vi "BStAT_(Singles).vi"() -> ()   [LabVIEW 2013]
uses:
  <vilib>/Utility/miscctls.llb/LVPositionTypeDef.ctl
  <vilib>/Utility/file.llb/Read From Spreadsheet File (DBL).vi
  <vilib>/Utility/file.llb/Write To Spreadsheet File (I64).vi
panel:
  out "framesPerSecond":u32
  out "serve to point":dbl[](array[numeric])
  in  "Word._Application":refnum<k7>
  out "p2y":dbl[](array[numeric])
  out "p1y":dbl[](array[numeric])
  out "point frames":dbl[](array[numeric])
  out "service frames":dbl[](array[numeric])
  out "comp_p1 2":dbl[](array[numeric])
  out "comp_p2 2":dbl[](array[numeric])
  out "comp_p2":dbl[](array[numeric])
  out "comp_p1":dbl[](array[numeric])
  out "game":i32[][](array[numeric])
  out "save2_data":dbl[][](array[numeric])
  out "save1_data":dbl[][](array[numeric])
  out "save2":i32[][](array[numeric])
  out "save1":i32[][](array[numeric])
  out "filedata in":dbl[][](array[numeric]) format="%0.3f"
  out "edited\nevents":dbl[][](array[numeric])
  out "edited to play":dbl[](array[numeric])
  out "P2 position":bool
  out "P1 position":bool
  out "p2code":i32
  out "p1code":i32
  out "frames":dbl[](array[numeric])
  out "Events":bool[](array[boolean])
  out "coded data":dbl[][](array[numeric])
  out "frame data":dbl[][](array[numeric])
  out "Score":dbl[][](array[numeric])
  out "OH":bool[](array[boolean])
  out "BH":bool[](array[boolean])
  out "FH":bool[](array[boolean])
  in  "stop":bool
  in  "Tab Control":enum32{"Coding", "Display"}(tab)
  in  "Drag control":u32(slide) min=400 max=3000 scale=0.0..37378.0
  in  "UNDO":bool
  out "Last coded":i32
  in  "Progress...":i32(slide) min=400 max=3000 scale=0.0..36584.0
  in  "1":bool
  in  "E2":bool
  in  "E1":bool
  in  "P2":i32
  in  "W2":bool
  in  "W1":bool
  in  "P1":i32
  in  "Pause 2":bool
  in  "F_Fr":bool
  in  "S_Fr":bool
  out "Video":T1(plugin-control)
  in  "START":bool
  in  "Video file":path caption="Open AVI file"
  in  "Save data":path caption="Save data to file"
  in  "Start Coding":bool
  out "F_frame":u32
  out "S_frame":u32
  in  "playback speed":dbl(slide) step=0.25 scale=0.25..2.0
  in  "fast forward":bool
  in  "TL 2":bool
  in  "BR 2":bool
  in  "BL 2":bool
  in  "BM 2":bool
  in  "CR  2":bool
  in  "CM 2":bool
  in  "CL 2":bool
  in  "TR 2":bool
  in  "TM 2":bool
  in  "TL 3":bool
  in  "BR 3":bool
  in  "BL 3":bool
  in  "BM 3":bool
  in  "CR  3":bool
  in  "CM 3":bool
  in  "CL 3":bool
  in  "TR 3":bool
  in  "TM 3":bool
  in  "Pause 1":bool
  out "coding":i32[][](array[numeric])
  in  "1 6":bool
  in  "2 6":bool
  in  "3 6":bool
  in  "4 6":bool
  in  "5 6":bool
  in  "6 6":bool
  in  "7 6":bool
  in  "8 6":bool
  in  "1 5":bool
  in  "2 5":bool
  in  "3 5":bool
  in  "4 5":bool
  in  "5 5":bool
  in  "6 5":bool
  in  "7 5":bool
  in  "8 5":bool
  in  "8 3":bool
  in  "7 3":bool
  in  "6 3":bool
  in  "5 3":bool
  in  "4 3":bool
  in  "3 3":bool
  in  "2 3":bool
  in  "1 3":bool
  in  "8 4":bool
  in  "7 4":bool
  in  "6 4":bool
  in  "5 4":bool
  in  "4 4":bool
  in  "3 4":bool
  in  "2 4":bool
  in  "1 4":bool
  in  "1 2":bool
  in  "2 2":bool
  in  "3 2":bool
  in  "4 2":bool
  in  "5 2":bool
  in  "6 2":bool
  in  "7 2":bool
  in  "8 2":bool
  in  "5":bool
  in  "6":bool
  in  "7":bool
  in  "8":bool
  in  "1":bool
  in  "2":bool
  in  "3":bool
  in  "4":bool
  in  "S2":bool
  in  "S1":bool
  in  "2":bool
  in  "3":bool
  in  "4":bool
  in  "Pause 3":bool
  in  "court":bool
  in  "Stop and save":bool
  out "Numeric":dbl format="%<%H:%M:%S>t"
  in  "play back":i32(slide)=1 min=0 max=7 scale=0.0..7.0
  out "DISP":T1(plugin-control)
  in  "Vid file":path caption="Open AVI file"
  in  "Data file":path caption="Read data from"
  in  "Tab Control 2":enum32{"Edit ", "Data Display", "Momentum"}(tab)
  in  "shots":u8(slide)=2 scale=0.0..5.0
  in  "point 2":bool
  in  "Rally":bool
  in  "Write VI":path caption="Write to AVI file"
  in  "before":u8(slide)=2
  in  "Playback Speed":dbl(slide)=1.0 min=0.25 max=30.0 step=0.25 scale=0.25..2.0
  in  "pause":bool
  in  "stop 2":bool
  in  "Playback\nscore":bool
  in  "P2 score":dbl
  in  "P1 score":dbl
  in  "error":bool
  in  "winner":bool
  in  "point 1":bool
  in  "player1":bool
  in  "player2":bool
  in  "1 7":bool
  in  "service2":bool
  in  "service1":bool
  in  "2 7":bool
  in  "3 7":bool
  in  "4 7":bool
  in  "TL":bool
  in  "BR":bool
  in  "BL":bool
  in  "BM":bool
  in  "CR":bool
  in  "CM":bool
  in  "CL":bool
  in  "TR":bool
  in  "TM":bool
  in  "FH 2":bool
  in  "BH 2":bool
  in  "ST":bool
  in  "CR 2":bool
  in  "lob":bool
  in  "clear":bool
  in  "drive":bool
  in  "smash":bool
  in  "defense":bool
  in  "chop":bool
  in  "drop":bool
  in  "net":bool
  in  "OH 2":bool
  in  "Play":bool
  in  "after":u8(slide)=2 scale=0.0..5.0
  in  "write file":bool
  out "Search events":i32(slide) caption="Scaning(events)..." min=400 max=3000 scale=0.0..903.0
  out "Search score":i32(slide) caption="Searching(score)..." min=400 max=3000 scale=0.0..1.0
  out "writing":i32(slide) caption="Writing..." min=400 max=3000 scale=0.0..7.0
  in  "3 shots":bool
  in  "Compare":bool
  in  "2":string(combo)="1"
  in  "1":string(combo)="1"
  in  "save2":string
  in  "save1":string
  in  "save2":bool
  in  "save1":bool
  in  "Percentage":bool
  in  "display\nselection":string(combo)="1"
  in  "To make white":enum32{""}(tab)
  out "player1 2":string[](array[string])
  out "player2 2":string[](array[string])
  out "P1graph":cluster{dbl[], "array":dbl[]}(graph)={[0.0, nan, 0.0, nan, 0.0, nan, 0.0, nan, 0.0, nan, 0.0, nan, 0.0, nan, 0.0, nan, 0.0], "array"=[1.0, 2.0, 3.0, 4.0, 5.0, 6.0, 7.0, 8.0, 9.0, 10.0, 11.0, 12.0, 13.0, 14.0, 15.0, 16.0, 17.0]}
  out "P2graph":cluster{dbl[], "array":dbl[]}(graph)={[0.0, nan, 0.0, nan, 0.0, nan, 0.0, nan, 0.0, nan, 0.0, nan, 0.0, nan, 0.0, nan, 0.0], "array"=[1.0, 2.0, 3.0, 4.0, 5.0, 6.0, 7.0, 8.0, 9.0, 10.0, 11.0, 12.0, 13.0, 14.0, 15.0, 16.0, 17.0]}
  out "W1/E1":string[](array[string])
  out "W2/E2":string[](array[string])
  out "W/E2":string[](array[string])=["Fore hand", "Back hand", "Over head", "", "Strainght", "Cross", "", "Lob", "Clear", "Drive", "Smash", "Defence", "Chop", "Drop", "Net"]
  out "W/E1":string[](array[string])=["Fore hand", "Back hand", "Over head", "", "Strainght", "Cross", "", "Lob", "Clear", "Drive", "Smash", "Defence", "Chop", "Drop", "Net"]
  out "player2_2":string[](array[string])
  out "player1_2":string[](array[string])
  out "Player 2":string[](array[string])=["Fore hand", "Back hand", "Over head", "", "Straight", "Cross", "", "Smash", "Defense", "Drive/Tap", "Lob", "Drop", "Chop", "Clear", "Net"]
  out "Player 2_2":string[](array[string])=["Fore hand", "Back hand", "Over head", "", "Strainght", "Cross", "", "Lob", "Clear", "Drive", "Smash", "Defence", "Chop", "Drop", "Net"]
  out "Player 1_2":string[](array[string])=["Fore hand", "Back hand", "Over head", "", "Strainght", "Cross", "", "Lob", "Clear", "Drive", "Smash", "Defence", "Chop", "Drop", "Net"]
  out "Player 1":string[](array[string])=["Fore hand", "Back hand", "Over head", "", "Straight", "Cross", "", "Smash", "Defense", "Drive/Tap", "Lob", "Drop", "Chop", "Clear", "Net"]
  out "p2 17":string
  out "p2 16":string
  out "p2 11":string
  out "p2 10":string
  out "p2 9":string
  out "p2 14":string
  out "p2 13":string
  out "p2 12":string
  out "p2 15":string
  out "p1 5":string
  out "p1 7":string
  out "p1 6":string
  out "p1 4":string
  out "p1 1":string
  out "p1 3":string
  out "p1 2":string
  out "p1 8":string
  out "p1 9":string
  in  "to make white 2":enum32{""}(tab)
  out "Shortest rally length(sec)":dbl format="%#_3g"
  out "Longest rally length(sec)":dbl format="%#_3g"
  out "momentum graph":cluster{dbl[], dbl[]}[](graph)
  out "Score":dbl[](array[numeric])
  out "Average rally length(sec)":dbl format="%#_3g"
  out "Rally length(sec)":dbl format="%#_3g"
  in  "edit video":bool
  in  "REPORT":bool
  # "Strategic Analysis Tool for Badminton"
  # "Forehand"
  # "Backhand"
  # "Overhead"
  # "Position"
  # "Straight"
  # "Cross"
  # "Straight"
  # "Cross"
  # "Straight"
  # "Cross"
  # "Smash"
  # "Defence"
  # "Drive/Tap"
  # "Lob"
  # "Drop"
  # "Chop"
  # "Player 2\n\nPlayer 1"
  # "Player 1\n\nPlayer 2"
  # "Clear"
  # "Net"
  # "Score"
  # "© 2012 National Sports Institute of Malaysia All Rights Reserved"
  # "© 2012 National Sports Institute of Malaysia All Rights Reserved"
  # "Shots to Playback"
  # "Score"
  # "Player"
  # "Position"
  # "Special Events"
  # "Playback interval (s)"
  # "to"
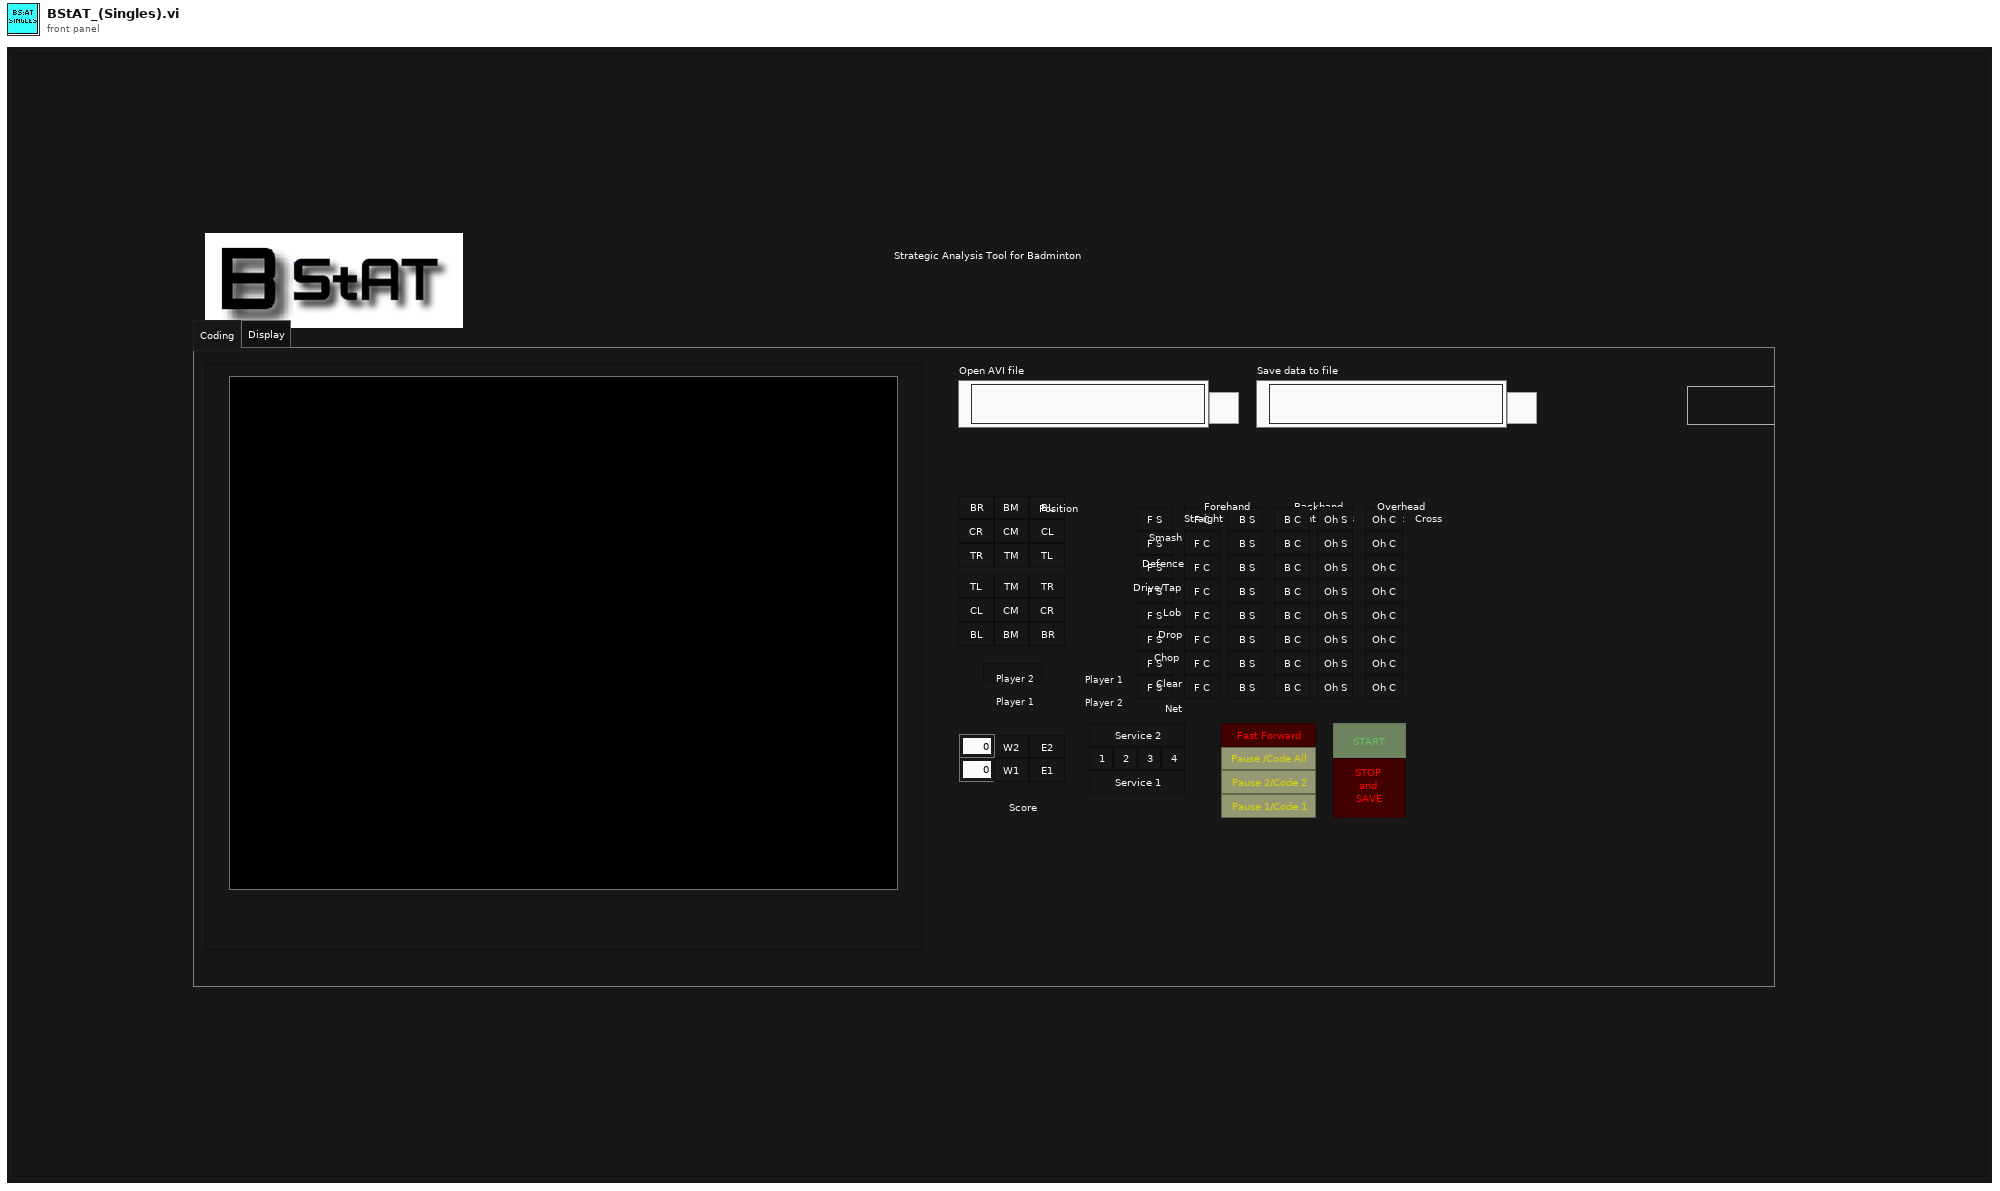
[diagram p1: front panel]
types:
  T1 = typedef "IMAQ Image.ctl" = refnum<image>
  T2 = enum8{"Enabled", "Disabled", "Disabled and Grayed Out"}
  T3 = enum16{"open", "replace", "create", "open or create", "replace or create", "replace or create with confirmation"}
  T4 = typedef "LVPositionTypeDef.ctl" = cluster{"Left":i32, "Top":i32}
  T5 = typedef "Image Type" = u32
  T6 = typedef "AviRefnum.ctl" = refnum<k1>
  T7 = cluster{"width":u32, "height":u32, "framesPerSecond":u32, "compressionFilter":string, "hasData":bool}
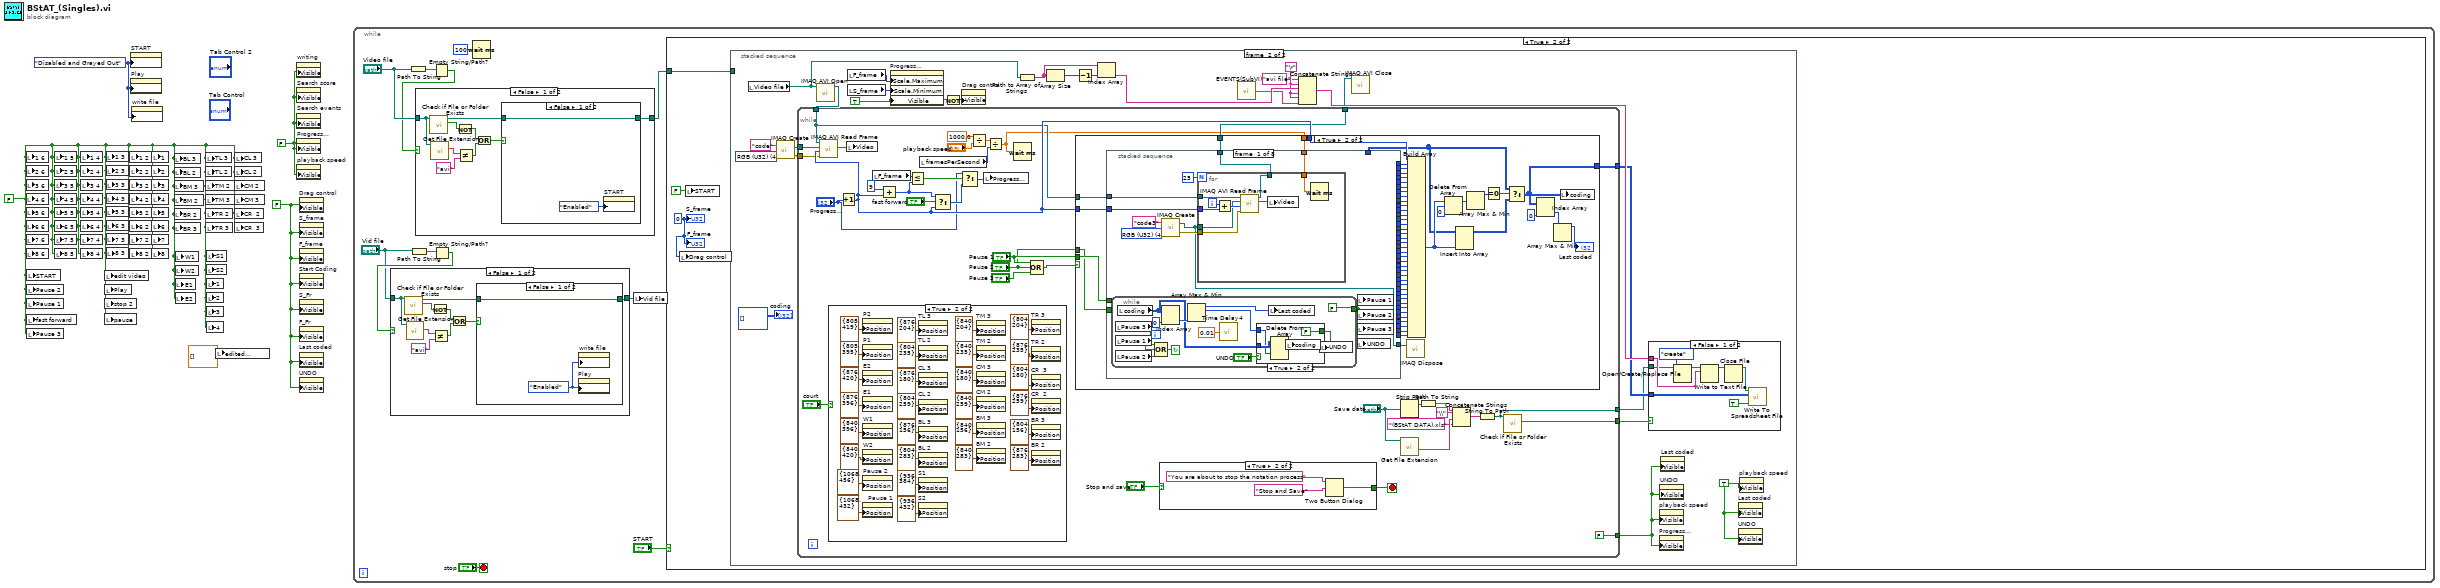
[diagram p0: block diagram]
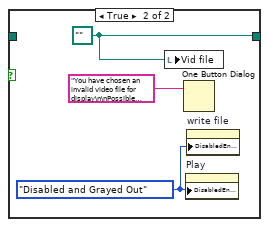
[diagram p2: hidden frame]
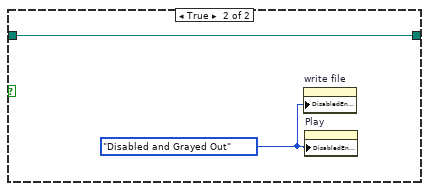
[diagram p3: hidden frame]
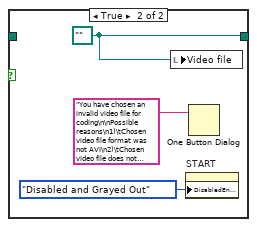
[diagram p4: hidden frame]
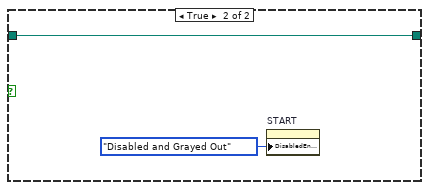
[diagram p5: hidden frame]
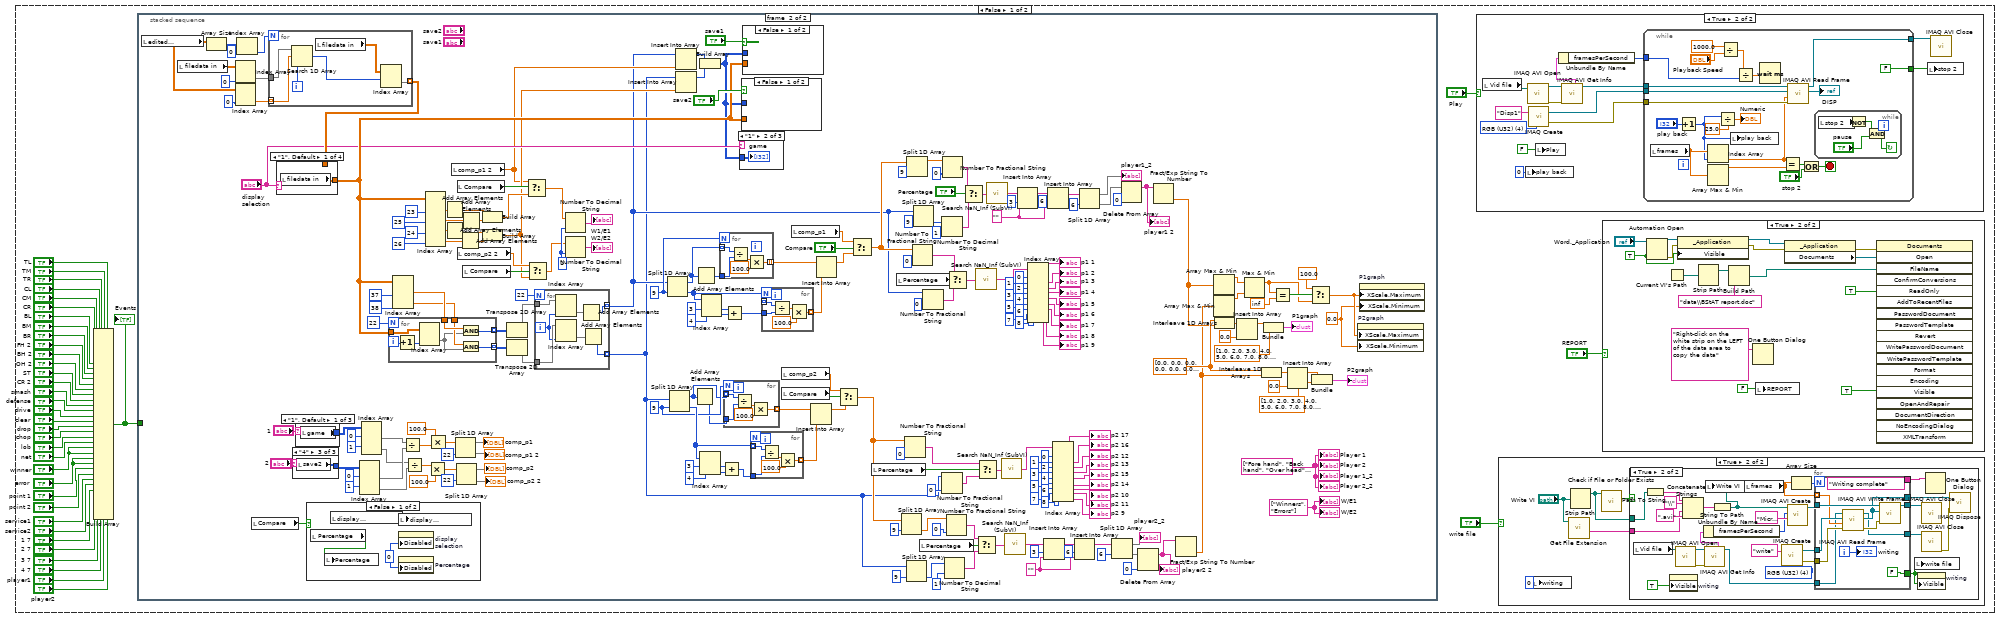
[diagram p6: hidden frame]
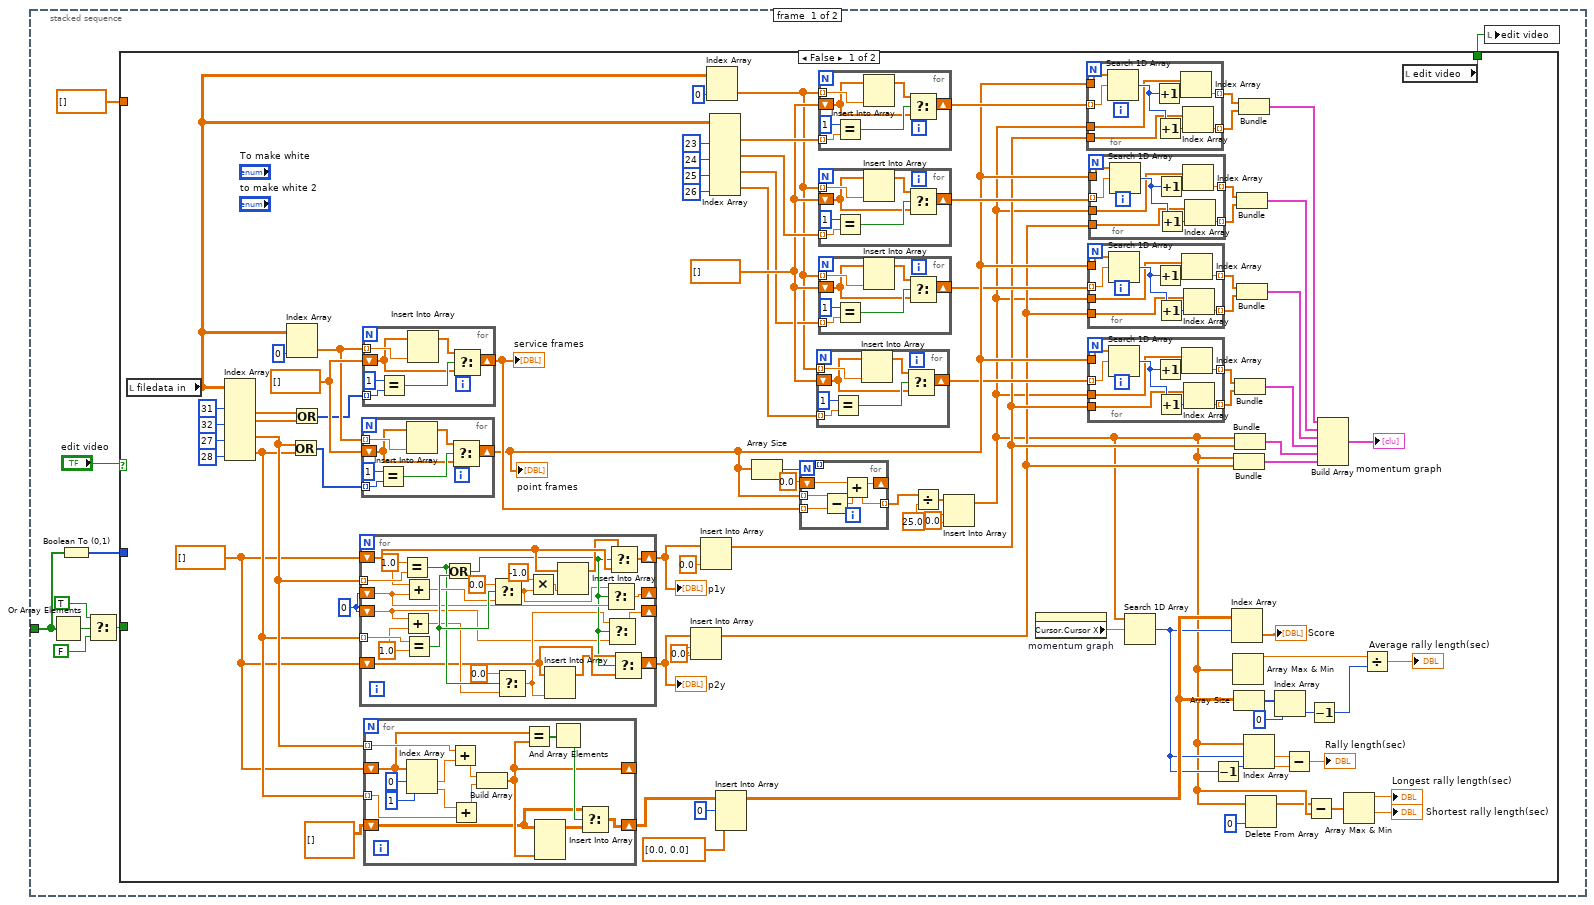
[diagram p8: hidden frame]
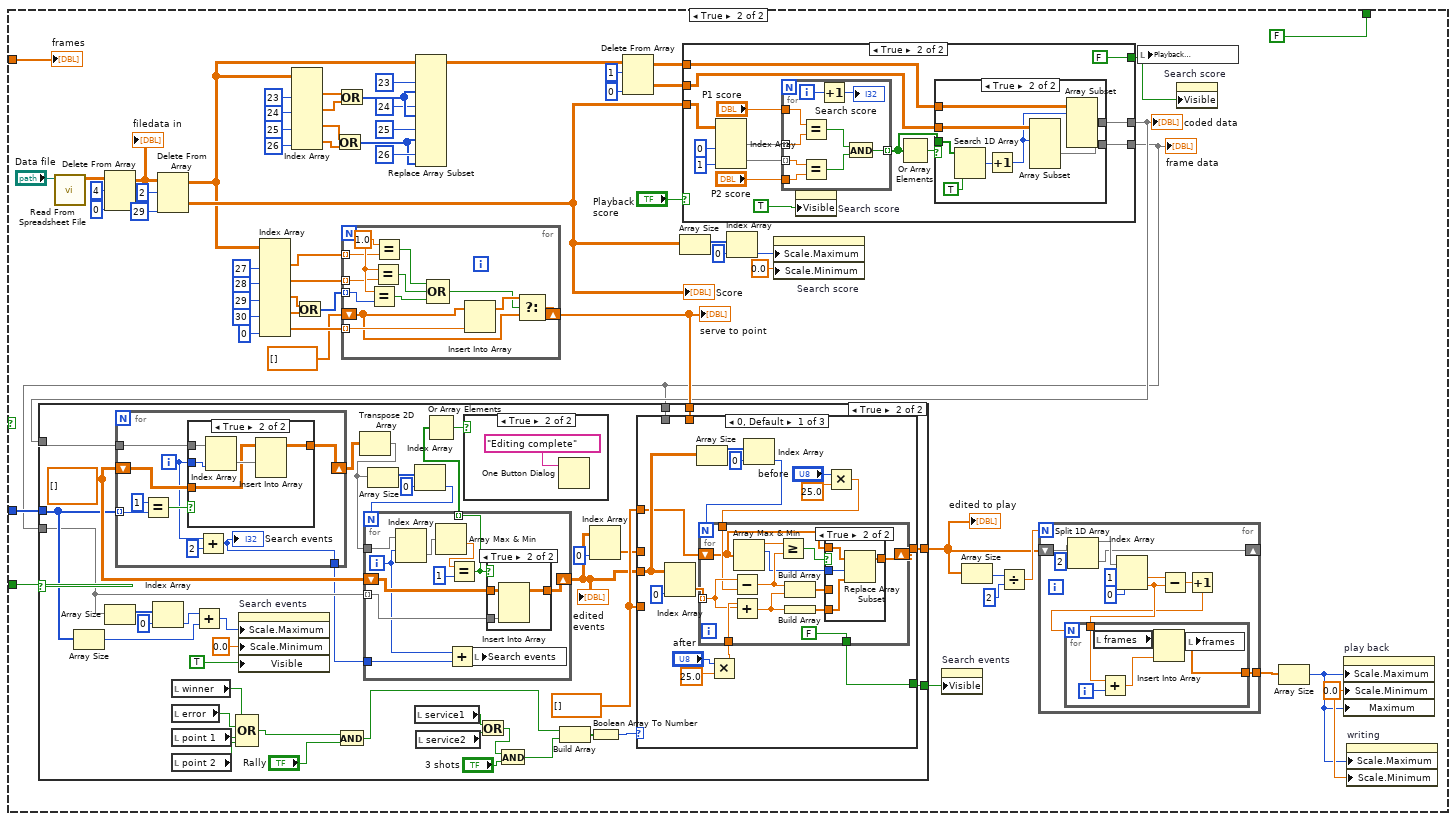
[diagram p9: hidden frame]
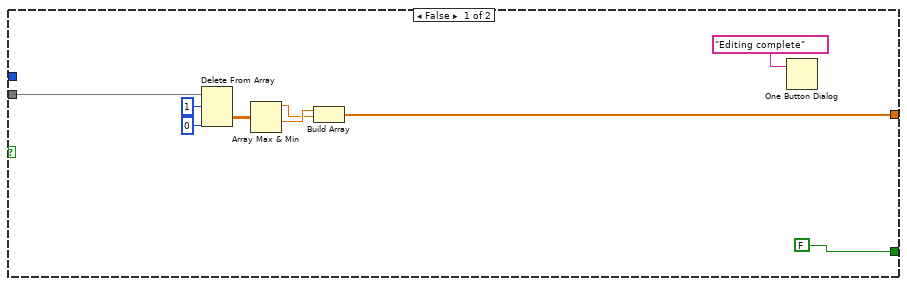
[diagram p10: hidden frame]
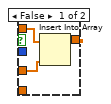
[diagram p11: hidden frame]
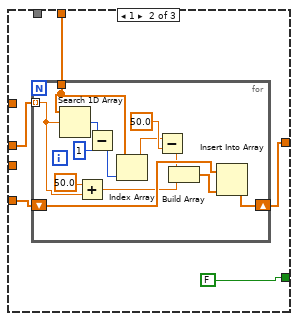
[diagram p12: hidden frame]
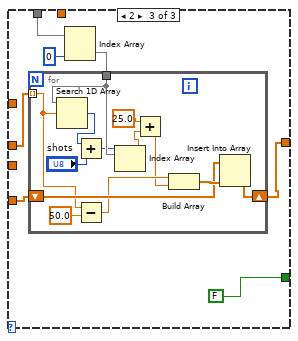
[diagram p13: hidden frame]
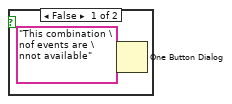
[diagram p14: hidden frame]
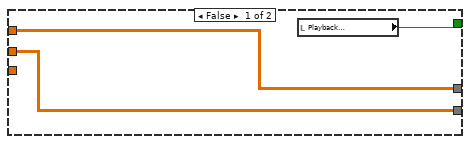
[diagram p17: hidden frame]
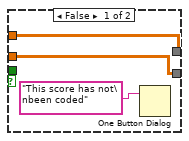
[diagram p18: hidden frame]
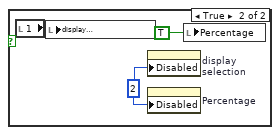
[diagram p19: hidden frame]
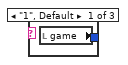
[diagram p20: hidden frame]
diagram:
  w1 = T2."Disabled and Grayed Out" ("Disabled")
  w3 = FALSE ("4 6")
  w2 = FALSE ("Visible")
  w4 = FALSE ("Visible")
  n1 = local write "1 6"(w3) -> ()
  n2 = local write "2 6"(w3) -> ()
  n3 = local write "3 6"(w3) -> ()
  n4 = local write "4 6"(w3) -> ()
  n5 = local write "5 6"(w3) -> ()
  n6 = local write "6 6"(w3) -> ()
  n7 = local write "7 6"(w3) -> ()
  n8 = local write "8 6"(w3) -> ()
  n9 = local write "START"(w3) -> ()
  n10 = local write "Pause 2"(w3) -> ()
  n11 = local write "Pause 1"(w3) -> ()
  n12 = local write "fast forward"(w3) -> ()
  n13 = local write "Pause 3"(w3) -> ()
  n14 = local write "1 5"(w3) -> ()
  n15 = local write "2 5"(w3) -> ()
  n16 = local write "3 5"(w3) -> ()
  n17 = local write "4 5"(w3) -> ()
  n18 = local write "5 5"(w3) -> ()
  n19 = local write "6 5"(w3) -> ()
  n20 = local write "7 5"(w3) -> ()
  n21 = local write "8 5"(w3) -> ()
  n22 = local write "1 4"(w3) -> ()
  n23 = local write "2 4"(w3) -> ()
  n24 = local write "3 4"(w3) -> ()
  n25 = local write "4 4"(w3) -> ()
  n26 = local write "5 4"(w3) -> ()
  n27 = local write "6 4"(w3) -> ()
  n28 = local write "7 4"(w3) -> ()
  n29 = local write "8 4"(w3) -> ()
  n30 = local write "edit video"(w3) -> ()
  n31 = local write "Play"(w3) -> ()
  n32 = local write "stop 2"(w3) -> ()
  n33 = local write "pause"(w3) -> ()
  n34 = local write "1 3"(w3) -> ()
  n35 = local write "2 3"(w3) -> ()
  n36 = local write "3 3"(w3) -> ()
  n37 = local write "4 3"(w3) -> ()
  n38 = local write "5 3"(w3) -> ()
  n39 = local write "6 3"(w3) -> ()
  n40 = local write "7 3"(w3) -> ()
  n41 = local write "8 3"(w3) -> ()
  n42 = local write "1 2"(w3) -> ()
  n43 = local write "2 2"(w3) -> ()
  n44 = local write "3 2"(w3) -> ()
  n45 = local write "4 2"(w3) -> ()
  n46 = local write "5 2"(w3) -> ()
  n47 = local write "6 2"(w3) -> ()
  n48 = local write "7 2"(w3) -> ()
  n49 = local write "8 2"(w3) -> ()
  n50 = property on="START" class="Bool (strict)"("DisabledEnum"=w1) -> ()  [unwired: 2 in, 2 out]
  n51 = property on="Play" class="Bool (strict)"("DisabledEnum"=w1) -> ()  [unwired: 2 in, 2 out]
  n52 = property on="write file" class="Bool (strict)"("DisabledEnum"=w1) -> ()  [unwired: 2 in, 2 out]
  n53 = local write "1"(w3) -> ()
  n54 = local write "2"(w3) -> ()
  n55 = local write "3"(w3) -> ()
  n56 = local write "4"(w3) -> ()
  n57 = local write "5"(w3) -> ()
  n58 = local write "6"(w3) -> ()
  n59 = local write "7"(w3) -> ()
  n60 = local write "8"(w3) -> ()
  n61 = local write "BL 3"(w3) -> ()
  n62 = local write "BL 2"(w3) -> ()
  n63 = local write "BM 3"(w3) -> ()
  n64 = local write "BM 2"(w3) -> ()
  n65 = local write "BR 2"(w3) -> ()
  n66 = local write "BR 3"(w3) -> ()
  n67 = local write "W1"(w3) -> ()
  n68 = local write "W2"(w3) -> ()
  n69 = local write "E1"(w3) -> ()
  n70 = local write "E2"(w3) -> ()
  n71 = local write "TL 3"(w3) -> ()
  n72 = local write "TL 2"(w3) -> ()
  n73 = local write "TM 2"(w3) -> ()
  n74 = local write "TM 3"(w3) -> ()
  n75 = local write "TR 2"(w3) -> ()
  n76 = local write "TR 3"(w3) -> ()
  n77 = local write "S1"(w3) -> ()
  n78 = local write "S2"(w3) -> ()
  n79 = local write "1"(w3) -> ()
  n80 = local write "2"(w3) -> ()
  n81 = local write "3"(w3) -> ()
  n82 = local write "4"(w3) -> ()
  n83 = local write "edited\nevents"(dbl[][] []) -> ()
  n84 = local write "CL 3"(w3) -> ()
  n85 = local write "CL 2"(w3) -> ()
  n86 = local write "CM 2"(w3) -> ()
  n87 = local write "CM 3"(w3) -> ()
  n88 = local write "CR  2"(w3) -> ()
  n89 = local write "CR  3"(w3) -> ()
  n90 = property on="writing" class="Slide (strict)"("Visible"=w4) -> ()  [unwired: 2 in, 2 out]
  n91 = property on="Search score" class="Slide (strict)"("Visible"=w4) -> ()  [unwired: 2 in, 2 out]
  n92 = property on="Search events" class="Slide (strict)"("Visible"=w4) -> ()  [unwired: 2 in, 2 out]
  n93 = property on="Progress..." class="Slide (strict)"("Visible"=w4) -> ()  [unwired: 2 in, 2 out]
  n94 = property on="playback speed" class="Slide (strict)"("Visible"=w4) -> ()  [unwired: 2 in, 2 out]
  n95 = property on="Drag control" class="Slide (strict)"("Visible"=w2) -> ()  [unwired: 2 in, 2 out]
  n96 = property on="S_frame" class="DigNum (strict)"("Visible"=w2) -> ()  [unwired: 2 in, 2 out]
  n97 = property on="F_frame" class="DigNum (strict)"("Visible"=w2) -> ()  [unwired: 2 in, 2 out]
  n98 = property on="Start Coding" class="Bool (strict)"("Visible"=w2) -> ()  [unwired: 2 in, 2 out]
  n99 = property on="S_Fr" class="Bool (strict)"("Visible"=w2) -> ()  [unwired: 2 in, 2 out]
  n100 = property on="F_Fr" class="Bool (strict)"("Visible"=w2) -> ()  [unwired: 2 in, 2 out]
  n101 = property on="Last coded" class="DigNum (strict)"("Visible"=w2) -> ()  [unwired: 2 in, 2 out]
  n102 = property on="UNDO" class="Bool (strict)"("Visible"=w2) -> ()  [unwired: 2 in, 2 out]
  n103 = while {
    stop <- "stop" stop-if-true
    n104 = Path To String(path="Video file") -> (string=w13:string)
    n105 = Path To String(path="Vid file") -> (string=w9:string)
    n106 = Empty String/Path?(string/path=w13) -> (empty?=w10:bool)
    n107 = case shown="False" w10 {
      tunnel: "Video file" -> [w41 w48]
      tunnel: [w35 w48] -> w11
      frame False {
        n108 = call <vilib>:"Check if File or Folder Exists.vi"("path"=w41) -> ("file or folder exists?"=w34:bool, "dup path"=w36:path)  [unwired: 8 in, 1 out]
        n109 = call <vilib>:"Get File Extension.vi"("file"=w41) -> ("lowercase file extension"=w40:string)  [unwired: 7 in, 3 out]
        n110 = Not(x=w34) -> (.not. x?=w33:bool)
        n111 = Not Equal?(x=w40, y="avi" ("lowercase file extension")) -> (x != y?=w38:bool)
        n112 = Or(x=w33, y=w38) -> (x .or. y?=w37:bool)
        n113 = case shown="False" w37 {
          tunnel: [w43 w46] -> w35
          tunnel: w36 -> [w43 _]
          frame False {
            n114 = property on="START" class="Bool (strict)"("DisabledEnum"=T2."Enabled" ("Disabled")) -> ()  [unwired: 2 in, 2 out]
          }
          frame True {
            w46 = path "" ("Video file")
            n115 = local write "Video file"(w46) -> ()
            n116 = property on="START" class="Bool (strict)"("DisabledEnum"=T2."Disabled and Grayed Out" ("Disabled")) -> ()  [unwired: 2 in, 2 out]
            n117 = One Button Dialog(message="You have chosen an invalid video file for coding\n\nPossible reasons\n1)\tChosen video file format was not AVI\n2)\tChosen video file does not exist") -> ()  [unwired: 1 in, 1 out]
          }
        }
      }
      frame True {
        n118 = property on="START" class="Bool (strict)"("DisabledEnum"=T2."Disabled and Grayed Out" ("Disabled")) -> ()  [unwired: 2 in, 2 out]
      }
    }
    n119 = Empty String/Path?(string/path=w9) -> (empty?=w8:bool)
    n120 = case shown="False" w8 {
      tunnel: "Vid file" -> [w25 w32]
      tunnel: [w19 w32] -> w6
      frame False {
        n121 = call <vilib>:"Check if File or Folder Exists.vi"("path"=w25) -> ("file or folder exists?"=w18:bool, "dup path"=w20:path)  [unwired: 8 in, 1 out]
        n122 = call <vilib>:"Get File Extension.vi"("file"=w25) -> ("lowercase file extension"=w24:string)  [unwired: 7 in, 3 out]
        n123 = Not(x=w18) -> (.not. x?=w17:bool)
        n124 = Not Equal?(x=w24, y="avi" ("lowercase file extension")) -> (x != y?=w22:bool)
        n125 = Or(x=w17, y=w22) -> (x .or. y?=w21:bool)
        n126 = case shown="False" w21 {
          tunnel: [w27 w29] -> w19
          tunnel: w20 -> [w27 _]
          frame False {
            w26 = T2."Enabled" ("Disabled")
            n127 = property on="Play" class="Bool (strict)"("DisabledEnum"=w26) -> ()  [unwired: 2 in, 2 out]
            n128 = property on="write file" class="Bool (strict)"("DisabledEnum"=w26) -> ()  [unwired: 2 in, 2 out]
          }
          frame True {
            w28 = T2."Disabled and Grayed Out" ("Disabled")
            w29 = path "" ("Video file")
            n129 = local write "Vid file"(w29) -> ()
            n130 = One Button Dialog(message="You have chosen an invalid video file for display\n\nPossible reasons\n1)\tChosen video file format was not AVI\n2)\tChosen video file does not exist") -> ()  [unwired: 1 in, 1 out]
            n131 = property on="Play" class="Bool (strict)"("DisabledEnum"=w28) -> ()  [unwired: 2 in, 2 out]
            n132 = property on="write file" class="Bool (strict)"("DisabledEnum"=w28) -> ()  [unwired: 2 in, 2 out]
          }
        }
      }
      frame True {
        w31 = T2."Disabled and Grayed Out" ("Disabled")
        n133 = property on="write file" class="Bool (strict)"("DisabledEnum"=w31) -> ()  [unwired: 2 in, 2 out]
        n134 = property on="Play" class="Bool (strict)"("DisabledEnum"=w31) -> ()  [unwired: 2 in, 2 out]
      }
    }
    n135 = Wait (ms)(milliseconds to wait=u32 100) -> ()  [unwired: 1 out]
    n136 = local write "Vid file"(w6) -> ()
    n137 = case shown="True" "START" {
      tunnel: w11 -> [_ w975]
      frame False {
        n138 = Build Array("TL", "TM", "TR", "CL", "CM", "CR", "BL", "BM", "BR", "FH 2", "BH 2", "OH 2", "ST", "CR 2", "smash", "defense", "drive", "clear", "drop", "chop", "lob", "net", "winner", "winner", "error", "error", "point 1", "point 2", "service1", "service2", "1 7", "2 7", "3 7", "4 7", "player1", "player2") -> (w61:bool[])
        "Events" <- w61
        n139 = stacked-sequence {
          tunnel: w61 -> [w108 _]
          frame #0 {
            n140 = Or Array Elements(Boolean array=w108) -> (logical OR=w111:bool)
            n141 = Boolean To (0,1)(Boolean=w108) -> (0, 1=w107:i16[])
            n142 = Select(t=TRUE, s=w111, f=FALSE) -> (s? t:f=w106:bool)
            n143 = case shown="False" "edit video" {
              tunnel: [w196 FALSE ("edit video")] -> w103
              tunnel: w107 -> [_ w325]
              tunnel: w106 -> [_ w364]
              tunnel: dbl[] [] ("edited\nto play 3") -> [_ w362]
              frame False {
                w152 = dbl[] []
                w186 = 0.0 ("new element/subarray")
                w185 = 0.0 ("new element/subarray")
                w184 = 0.0 ("new element/subarray")
                w134 = dbl[] []
                w137 = 0 ("disabled index (col)")
                w177 = dbl[] []
                n144 = local read "filedata in"() -> (w153:dbl[][])
                n145 = Index Array(array=w153, index (col) #1=31 ("length"), index (col) #2=32 ("disabled index (col)"), index (col) #3=27 ("index (col)"), index (col) #4=28 ("index (col)")) -> (element #1=w169:dbl[], element #2=w170:dbl[], element #3=w136:dbl[], element #4=w135:dbl[])  [unwired: 4 in]
                n146 = Index Array(array=w153, index (col)=0 ("disabled index (col)")) -> (element=w176:dbl[])  [unwired: 1 in]
                n147 = Or(x=w136, y=w135) -> (x .or. y?=w175:i32[])
                n148 = Or(x=w169, y=w170) -> (x .or. y?=w172:i32[])
                n149 = for {
                  shift-right: [w205] -> _
                  shift-left: w137 -> [w204]
                  shift-right: [w201] -> _
                  shift-left: w137 -> [w200]
                  shift-right: [w210] -> w132
                  shift-left: w134 -> [w209]
                  shift-right: [w216] -> w133
                  shift-left: w134 -> [w207]
                  tunnel: w135 -> [w213] mode=indexing
                  tunnel: w136 -> [w221] mode=indexing
                  w212 = 1.0 ("x")
                  w218 = 1.0 ("x")
                  n150 = Equal?(x=w218, y=w221) -> (x = y?=w214:bool)
                  n151 = Add(x=w200, y=w212) -> (x+y=w211:dbl)
                  n152 = Add(x=w218, y=w204) -> (x+y=w217:dbl)
                  n153 = Equal?(x=w213, y=w212) -> (x = y?=w220:bool)
                  n154 = Or(x=w214, y=w220) -> (x .or. y?=w203:bool)
                  n155 = Select(t=0.0, s=w220, f=w217) -> (s? t:f=w197:dbl)
                  n156 = Select(t=0.0, s=w214, f=w211) -> (s? t:f=w202:dbl)
                  n157 = Multiply(x=-1.0 ("y"), y=w197) -> (x*y=w199:dbl)
                  n158 = Insert Into Array(array=w207, new element=w202) -> (w206:dbl[])  [unwired: 1 in]
                  n159 = Insert Into Array(array=w209, new element=w199) -> (w208:dbl[])  [unwired: 1 in]
                  n160 = Select(t=w197, s=w203, f=w204) -> (s? t:f=w205:dbl)
                  n161 = Select(t=w202, s=w203, f=w200) -> (s? t:f=w201:dbl)
                  n162 = Select(t=w208, s=w203, f=w209) -> (s? t:f=w210:dbl[])
                  n163 = Select(t=w206, s=w203, f=w207) -> (s? t:f=w216:dbl[])
                }
                "p1y" <- w132
                "p2y" <- w133
                n164 = for {
                  tunnel: w175 -> [w313] mode=indexing
                  tunnel: w176 -> [w309] mode=indexing
                  shift-right: [w308] -> w148
                  shift-left: w177 -> [w307]
                  n165 = Equal?(x=1, y=w313) -> (x = y?=w311:bool)
                  n166 = Insert Into Array(array=w307, new element=w309) -> (w310:dbl[])  [unwired: 1 in]
                  n167 = Select(t=w310, s=w311, f=w307) -> (s? t:f=w308:dbl[])
                }
                "point frames" <- w148
                n168 = for {
                  tunnel: w172 -> [w320] mode=indexing
                  tunnel: w176 -> [w316] mode=indexing
                  shift-right: [w315] -> w179
                  shift-left: w177 -> [w314]
                  n169 = Equal?(x=1, y=w320) -> (x = y?=w318:bool)
                  n170 = Insert Into Array(array=w314, new element=w316) -> (w317:dbl[])  [unwired: 1 in]
                  n171 = Select(t=w317, s=w318, f=w314) -> (s? t:f=w315:dbl[])
                }
                "service frames" <- w179
                n172 = for {
                  tunnel: w136 -> [w297] mode=indexing
                  tunnel: w135 -> [w293] mode=indexing
                  shift-right: [w289] -> _
                  shift-left: w134 -> [w292]
                  shift-right: [w287] -> w191
                  shift-left: dbl[][] [] -> [w286]
                  n173 = Index Array(array=w292, index #1=0 ("index"), index #2=1 ("index")) -> (element #1=w298:dbl, element #2=w296:dbl)
                  n174 = Add(x=w297, y=w298) -> (x+y=w295:dbl)
                  n175 = Add(x=w296, y=w293) -> (x+y=w294:dbl)
                  n176 = Build Array(w295, w294) -> (w289:dbl[])
                  n177 = Equal?(x=w292, y=w289) -> (x = y?=w291:bool[])
                  n178 = Insert Into Array(array=w286, new element=w289) -> (w288:dbl[][])  [unwired: 2 in]
                  n179 = And Array Elements(Boolean array=w291) -> (logical AND=w290:bool)
                  n180 = Select(t=w286, s=w290, f=w288) -> (s? t:f=w287:dbl[][])
                }
                n181 = Insert Into Array(array=w133, index=w185, new element=w185) -> (w130:dbl[])
                n182 = Insert Into Array(array=w132, index=w186, new element=w186) -> (w131:dbl[])
                n183 = Index Array(array=w153, index (col)=0 ("disabled index (col)")) -> (element=w149:dbl[])  [unwired: 1 in]
                n184 = Index Array(array=w153, index (col) #1=23 ("disabled index (col)"), index (col) #2=24 ("index (col)"), index (col) #3=25 ("index (col)"), index (col) #4=26 ("index (col)")) -> (element #1=w162:dbl[], element #2=w163:dbl[], element #3=w151:dbl[], element #4=w150:dbl[])  [unwired: 4 in]
                n185 = Insert Into Array(array=w191, index (row)=0, new element=dbl[] [0.0, 0.0] ("new element/subarray")) -> (w129:dbl[][])  [unwired: 1 in]
                n186 = Array Size(array=w148) -> (size(s)=w178:i32)
                n187 = for {
                  N: w178 -> [w301]
                  tunnel: w148 -> [w306] mode=indexing
                  tunnel: w179 -> [w305] mode=indexing
                  tunnel: [w302] -> w188 mode=indexing
                  shift-right: [w302] -> _
                  shift-left: 0.0 -> [w303]
                  tunnel: [w301] -> _ mode=indexing
                  n188 = Subtract(x=w306, y=w305) -> (x-y=w304:dbl)
                  n189 = Add(x=w303, y=w304) -> (x+y=w302:dbl)
                }
                n190 = for {
                  tunnel: w150 -> [w246] mode=indexing
                  tunnel: w149 -> [w242] mode=indexing
                  shift-right: [w241] -> w146
                  shift-left: w152 -> [w240]
                  n191 = Equal?(x=1, y=w246) -> (x = y?=w244:bool)
                  n192 = Insert Into Array(array=w240, new element=w242) -> (w243:dbl[])  [unwired: 1 in]
                  n193 = Select(t=w243, s=w244, f=w240) -> (s? t:f=w241:dbl[])
                }
                n194 = for {
                  tunnel: w162 -> [w285] mode=indexing
                  tunnel: w149 -> [w281] mode=indexing
                  shift-right: [w280] -> w159
                  shift-left: w152 -> [w279]
                  n195 = Equal?(x=1, y=w285) -> (x = y?=w283:bool)
                  n196 = Insert Into Array(array=w279, new element=w281) -> (w282:dbl[])  [unwired: 1 in]
                  n197 = Select(t=w282, s=w283, f=w279) -> (s? t:f=w280:dbl[])
                }
                n198 = for {
                  tunnel: w163 -> [w278] mode=indexing
                  tunnel: w149 -> [w274] mode=indexing
                  shift-right: [w273] -> w164
                  shift-left: w152 -> [w272]
                  n199 = Equal?(x=1, y=w278) -> (x = y?=w276:bool)
                  n200 = Insert Into Array(array=w272, new element=w274) -> (w275:dbl[])  [unwired: 1 in]
                  n201 = Select(t=w275, s=w276, f=w272) -> (s? t:f=w273:dbl[])
                }
                n202 = for {
                  tunnel: w151 -> [w253] mode=indexing
                  tunnel: w149 -> [w249] mode=indexing
                  shift-right: [w248] -> w147
                  shift-left: w152 -> [w247]
                  n203 = Equal?(x=1, y=w253) -> (x = y?=w251:bool)
                  n204 = Insert Into Array(array=w247, new element=w249) -> (w250:dbl[])  [unwired: 1 in]
                  n205 = Select(t=w250, s=w251, f=w247) -> (s? t:f=w248:dbl[])
                }
                n206 = Divide(x=w188, y=25.0 ("new element/subarray")) -> (x/y=w187:dbl[])
                n207 = Insert Into Array(array=w187, index=w184, new element=w184) -> (w116:dbl[])
                n208 = property on="momentum graph" class="XYGraph (strict)"() -> ("Cursor.Cursor X"=w194:dbl)  [unwired: 2 in, 2 out]
                n209 = for {
                  tunnel: w159 -> [w271] mode=indexing
                  tunnel: w148 -> [w270]
                  tunnel: [w268] -> w160 mode=indexing
                  tunnel: [w265] -> w161 mode=indexing
                  tunnel: w116 -> [w264]
                  tunnel: w131 -> [w263]
                  n210 = Search 1D Array(1D array=w270, element=w271) -> (index of element=w266:i32)  [unwired: 1 in]
                  n211 = Increment(x=w266) -> (x+1=w269:i32)
                  n212 = Increment(x=w266) -> (x+1=w267:i32)
                  n213 = Index Array(array=w264, index=w269) -> (element=w268:dbl)
                  n214 = Index Array(array=w263, index=w267) -> (element=w265:dbl)
                }
                n215 = for {
                  tunnel: w147 -> [w239] mode=indexing
                  tunnel: w148 -> [w238]
                  tunnel: [w236] -> w145 mode=indexing
                  tunnel: [w233] -> w144 mode=indexing
                  tunnel: w116 -> [w232]
                  tunnel: w130 -> [w231]
                  n216 = Search 1D Array(1D array=w238, element=w239) -> (index of element=w234:i32)  [unwired: 1 in]
                  n217 = Increment(x=w234) -> (x+1=w237:i32)
                  n218 = Increment(x=w234) -> (x+1=w235:i32)
                  n219 = Index Array(array=w232, index=w237) -> (element=w236:dbl)
                  n220 = Index Array(array=w231, index=w235) -> (element=w233:dbl)
                }
                n221 = for {
                  tunnel: w146 -> [w230] mode=indexing
                  tunnel: w148 -> [w229]
                  tunnel: [w227] -> w143 mode=indexing
                  tunnel: [w224] -> w142 mode=indexing
                  tunnel: w116 -> [w223]
                  tunnel: w131 -> [w222]
                  n222 = Search 1D Array(1D array=w229, element=w230) -> (index of element=w225:i32)  [unwired: 1 in]
                  n223 = Increment(x=w225) -> (x+1=w228:i32)
                  n224 = Increment(x=w225) -> (x+1=w226:i32)
                  n225 = Index Array(array=w223, index=w228) -> (element=w227:dbl)
                  n226 = Index Array(array=w222, index=w226) -> (element=w224:dbl)
                }
                n227 = for {
                  tunnel: w164 -> [w262] mode=indexing
                  tunnel: w148 -> [w261]
                  tunnel: [w259] -> w165 mode=indexing
                  tunnel: [w256] -> w166 mode=indexing
                  tunnel: w116 -> [w255]
                  tunnel: w130 -> [w254]
                  n228 = Search 1D Array(1D array=w261, element=w262) -> (index of element=w257:i32)  [unwired: 1 in]
                  n229 = Increment(x=w257) -> (x+1=w260:i32)
                  n230 = Increment(x=w257) -> (x+1=w258:i32)
                  n231 = Index Array(array=w255, index=w260) -> (element=w259:dbl)
                  n232 = Index Array(array=w254, index=w258) -> (element=w256:dbl)
                }
                n233 = Search 1D Array(1D array=w116, element=w194) -> (index of element=w121:i32)  [unwired: 1 in]
                n234 = Decrement(x=w121) -> (x-1=w122:i32)
                n235 = Index Array(array=w129, index (row)=w121) -> (element=→"Score":dbl[])  [unwired: 1 in]
                n236 = Array Max & Min(array=w116) -> (max value=w125:dbl)  [unwired: 3 out]
                n237 = Bundle(w116, w130) -> (w180:cluster{dbl[], dbl[]})  [unwired: 1 in]
                n238 = Array Size(array=w129) -> (size(s)=w128:i32[])
                n239 = Bundle(w143, w142) -> (w138:cluster{dbl[], dbl[]})  [unwired: 1 in]
                n240 = Bundle(w116, w131) -> (w181:cluster{dbl[], dbl[]})  [unwired: 1 in]
                n241 = Bundle(w165, w166) -> (w140:cluster{dbl[], dbl[]})  [unwired: 1 in]
                n242 = Bundle(w145, w144) -> (w139:cluster{dbl[], dbl[]})  [unwired: 1 in]
                n243 = Bundle(w160, w161) -> (w141:cluster{dbl[], dbl[]})  [unwired: 1 in]
                n244 = Index Array(array=w116, index #1=w121, index #2=w122) -> (element #1=w119:dbl, element #2=w120:dbl)
                n245 = Delete From Array(array=w116, index=0) -> (array with subset deleted=w115:dbl[])  [unwired: 1 in, 1 out]
                n246 = Index Array(array=w128, index=0) -> (element=w126:i32)
                n247 = Subtract(x=w119, y=w120) -> (x-y=→"Rally length(sec)":dbl)
                n248 = Subtract(x=w115, y=w116) -> (x-y=w114:dbl[])
                n249 = Decrement(x=w126) -> (x-1=w124:i32)
                n250 = Build Array(w141, w140, w139, w138, w181, w180) -> (→"momentum graph":cluster{dbl[], dbl[]}[])
                n251 = Array Max & Min(array=w114) -> (max value=→"Longest rally length(sec)":dbl, min value=→"Shortest rally length(sec)":dbl)  [unwired: 2 out]
                n252 = Divide(x=w125, y=w124) -> (x/y=→"Average rally length(sec)":dbl)
                n253 = local read "edit video"() -> (w196:bool)
              }
              frame True {
                w360 = 0.0 ("Scale.Range:Minimum")
                n254 = call-poly <vilib>:"Read From Spreadsheet File.vi"("file path (dialog if empty)"="Data file") -> ("all rows"=w378:dbl[][])  [unwired: 6 in, 4 out]
                n255 = Delete From Array(array=w378, length=4, index (row)=0) -> (array with subset deleted=w357:dbl[][])  [unwired: 1 in, 1 out]
                "filedata in" <- w357
                n256 = Delete From Array(array=w357, length=2, index (col)=29 ("disabled index (col)")) -> (deleted portion=w369:dbl[][], array with subset deleted=w324:dbl[][])  [unwired: 1 in]
                "Score" <- w369
                n257 = Index Array(array=w324, index (col) #1=27 ("disabled index (col)"), index (col) #2=28 ("index (col)"), index (col) #3=29 ("index (col)"), index (col) #4=30 ("index (col)"), index (col) #5=0 ("index (col)")) -> (element #1=w331:dbl[], element #2=w332:dbl[], element #3=w330:dbl[], element #4=w329:dbl[], element #5=w334:dbl[])  [unwired: 5 in]
                n258 = Index Array(array=w324, index (col) #1=23 ("disabled index (col)"), index (col) #2=24 ("index (col)"), index (col) #3=25 ("index (col)"), index (col) #4=26 ("index (col)")) -> (element #1=w352:dbl[], element #2=w351:dbl[], element #3=w350:dbl[], element #4=w349:dbl[])  [unwired: 4 in]
                n259 = Or(x=w330, y=w329) -> (x .or. y?=w333:i32[])
                n260 = Or(x=w350, y=w349) -> (x .or. y?=w343:i32[])
                n261 = Or(x=w352, y=w351) -> (x .or. y?=w348:i32[])
                n262 = for {
                  tunnel: w331 -> [w384] mode=indexing
                  tunnel: w334 -> [w388] mode=indexing
                  tunnel: w333 -> [w382] mode=indexing
                  tunnel: w332 -> [w383] mode=indexing
                  shift-right: [w390] -> w328
                  shift-left: dbl[] [] -> [w387]
                  w389 = 1.0 ("x")
                  n263 = Equal?(x=w389, y=w382) -> (x = y?=w391:bool)
                  n264 = Equal?(x=w389, y=w383) -> (x = y?=w392:bool)
                  n265 = Equal?(x=w389, y=w384) -> (x = y?=w393:bool)
                  n266 = Compound Arithmetic op=OR(w393, w392, w391) -> (w385:bool)
                  n267 = Insert Into Array(array=w387, new element=w388) -> (w386:dbl[])  [unwired: 1 in]
                  n268 = Select(t=w386, s=w385, f=w387) -> (s? t:f=w390:dbl[])
                }
                "serve to point" <- w328
                n269 = Replace Array Subset(array=w324, new element #1=w348, index (col) #1=23 ("disabled index (col)"), new element #2=w348, index (col) #2=24 ("index (col)"), new element #3=w343, index (col) #3=25 ("index (col)"), new element #4=w343, index (col) #4=26 ("index (col)")) -> (w323:dbl[][])  [unwired: 4 in]
                n270 = Delete From Array(array=w323, length=1, index (col)=0 ("disabled index (col)")) -> (deleted portion=w372:dbl[][], array with subset deleted=w373:dbl[][])  [unwired: 1 in]
                n271 = Array Size(array=w369) -> (size(s)=w370:i32[])
                n272 = case shown="True" "Playback\nscore" {
                  tunnel: w373 -> [w566 w573]
                  tunnel: w372 -> [w565 w572]
                  tunnel: w369 -> [_ w582]
                  tunnel: [w567 FALSE ("element")] -> w366
                  tunnel: [w565 w570] -> w322
                  tunnel: [w566 w569] -> w327
                  frame False {
                    n273 = local read "Playback\nscore"() -> (w567:bool)
                  }
                  frame True {
                    n274 = Index Array(array=w582, index (col) #1=0 ("disabled index (col)"), index (col) #2=1 ("index (col)")) -> (element #1=w579:dbl[], element #2=w578:dbl[])  [unwired: 2 in]
                    n275 = for {
                      tunnel: w579 -> [w602] mode=indexing
                      tunnel: w578 -> [w600] mode=indexing
                      tunnel: "P1 score" -> [w601]
                      tunnel: "P2 score" -> [w599]
                      tunnel: [w597] -> w574 mode=indexing
                      i -> [w596]
                      n276 = Equal?(x=w601, y=w602) -> (x = y?=w598:bool)
                      n277 = Equal?(x=w600, y=w599) -> (x = y?=w594:bool)
                      n278 = Increment(x=w596) -> (x+1=→"Search score":i32)
                      n279 = And(x=w598, y=w594) -> (x .and. y?=w597:bool)
                    }
                    n280 = property on="Search score" class="Slide (strict)"("Visible"=TRUE) -> ()  [unwired: 2 in, 2 out]
                    n281 = Or Array Elements(Boolean array=w574) -> (logical OR=w575:bool)
                    n282 = case shown="True" w575 {
                      tunnel: w574 -> [_ w593]
                      tunnel: w573 -> [w585 w591]
                      tunnel: w572 -> [w584 w590]
                      tunnel: [w585 w589] -> w569
                      tunnel: [w584 w588] -> w570
                      frame False {
                        n283 = One Button Dialog(message="This score has not\nbeen coded") -> ()  [unwired: 1 in, 1 out]
                      }
                      frame True {
                        n284 = Search 1D Array(1D array=w593, element=TRUE) -> (index of element=w587:i32)  [unwired: 1 in]
                        n285 = Increment(x=w587) -> (x+1=w586:i32)
                        n286 = Array Subset(array=w590, index (row)=w586) -> (w588:dbl[][])  [unwired: 3 in]
                        n287 = Array Subset(array=w591, index (row)=w586) -> (w589:dbl[][])  [unwired: 3 in]
                      }
                    }
                  }
                }
                "frame data" <- w322
                "coded data" <- w327
                n288 = case shown="True" w364 {
                  tunnel: w327 -> [_ w459]
                  tunnel: w325 -> [_ w450]
                  tunnel: w322 -> [w413 w447]
                  tunnel: [w416 w440] -> w341
                  tunnel: [FALSE ("Visible") w439] -> w340
                  tunnel: w328 -> [_ w437]
                  tunnel: w322 -> [_ w433]
                  frame False {
                    n289 = Delete From Array(array=w413, length=1, index (col)=0 ("disabled index (col)")) -> (deleted portion=w412:dbl[][])  [unwired: 1 in, 1 out]
                    n290 = Array Max & Min(array=w412) -> (max value=w414:dbl, min value=w415:dbl)  [unwired: 2 out]
                    n291 = Build Array(w415, w414) -> (w416:dbl[])
                    n292 = One Button Dialog(message="Editing complete") -> ()  [unwired: 1 in, 1 out]
                  }
                  frame True {
                    w438 = dbl[] []
                    w451 = dbl[][] []
                    n293 = Array Size(array=w450) -> (size(s)=w444:i32)
                    n294 = Array Size(array=w447) -> (size(s)=w448:i32[])
                    n295 = for {
                      tunnel: w450 -> [w558] mode=indexing
                      tunnel: w459 -> [w555]
                      shift-right: [w554] -> w458
                      shift-left: w451 -> [w553]
                      tunnel: [w550] -> w442
                      i -> [w552]
                      n296 = Equal?(x=i16 1, y=w558) -> (x = y?=w556:bool)
                      n297 = case shown="True" w556 {
                        tunnel: w552 -> [_ w564]
                        tunnel: w555 -> [_ w563]
                        tunnel: [w559 w561] -> w554
                        tunnel: w553 -> [w559 w560]
                        frame False {
                        }
                        frame True {
                          n298 = Index Array(array=w563, index (col)=w564) -> (element=w562:dbl[])  [unwired: 1 in]
                          n299 = Insert Into Array(array=w560, new element=w562) -> (w561:dbl[][])  [unwired: 2 in]
                        }
                      }
                      n300 = Add(x=w552, y=2) -> (x+y=w550:i32)
                      "Search events" <- w550
                    }
                    n301 = Index Array(array=w448, index=0) -> (element=w443:i32)
                    n302 = local read "winner"() -> (w421:bool)
                    n303 = local read "error"() -> (w422:bool)
                    n304 = local read "point 1"() -> (w423:bool)
                    n305 = local read "point 2"() -> (w424:bool)
                    n306 = Add(x=w443, y=w444) -> (x+y=w446:i32)
                    n307 = Compound Arithmetic op=OR(w421, w422, w423, w424) -> (w420:bool)
                    n308 = property on="Search events" class="Slide (strict)"("Scale.Maximum"=w446, "Scale.Minimum"=0.0 ("Scale.Range:Minimum"), "Visible"=TRUE) -> ()  [unwired: 2 in, 2 out]
                    n309 = And(x=w420, y="Rally") -> (x .and. y?=w419:bool)
                    n310 = Transpose 2D Array(2D array=w458) -> (transposed array=w454:dbl[][])
                    n311 = Array Size(array=w454) -> (size(s)=w457:i32[])
                    n312 = Index Array(array=w457, index=0) -> (element=w455:i32)
                    n313 = for {
                      N: w455 -> [_]
                      tunnel: w447 -> [w543] mode=indexing
                      shift-right: [w542] -> w436
                      shift-left: w451 -> [w544]
                      tunnel: w454 -> [w541]
                      tunnel: [w538] -> w453 mode=indexing
                      tunnel: w442 -> [w535]
                      i -> [w536]
                      n314 = Index Array(array=w541, index (row)=w536) -> (element=w540:dbl[])  [unwired: 1 in]
                      n315 = Array Max & Min(array=w540) -> (min value=w539:dbl)  [unwired: 3 out]
                      n316 = Add(x=w536, y=w535) -> (x+y=w537:i32)
                      n317 = Equal?(x=w539, y=1) -> (x = y?=w538:bool)
                      n318 = local write "Search events"(w537) -> ()
                      n319 = case shown="True" w538 {
                        tunnel: w544 -> [w546 w549]
                        tunnel: w543 -> [_ w548]
                        tunnel: [w546 w547] -> w542
                        frame False {
                        }
                        frame True {
                          n320 = Insert Into Array(array=w549, new element=w548) -> (w547:dbl[][])  [unwired: 2 in]
                        }
                      }
                    }
                    "edited\nevents" <- w436
                    n321 = local read "service1"() -> (w427:bool)
                    n322 = local read "service2"() -> (w428:bool)
                    n323 = Or Array Elements(Boolean array=w453) -> (logical OR=w452:bool)
                    n324 = case shown="True" w452 {
                      frame False {
                        n325 = One Button Dialog(message="This combination \nof events are \nnot available") -> ()  [unwired: 1 in, 1 out]
                      }
                      frame True {
                        n326 = One Button Dialog(message="Editing complete") -> ()  [unwired: 1 in, 1 out]
                      }
                    }
                    n327 = Or(x=w427, y=w428) -> (x .or. y?=w430:bool)
                    n328 = And(x=w430, y="3 shots") -> (x .and. y?=w426:bool)
                    n329 = Build Array(w419, w426) -> (w432:bool[])
                    n330 = Index Array(array=w436, index (col)=0 ("disabled index (col)")) -> (element=w434:dbl[])  [unwired: 1 in]
                    n331 = Boolean Array To Number(Boolean array=w432) -> (number=w431:u32)
                    n332 = case shown="0, Default" w431 {
                      tunnel: w436 -> [w463 _ _]
                      tunnel: [w462 w497 w513] -> w440
                      tunnel: [w461 FALSE ("Visible") FALSE ("Visible")] -> w439
                      tunnel: w438 -> [w460 _ _]
                      tunnel: w438 -> [_ w499 w517]
                      tunnel: w437 -> [_ w498 _]
                      tunnel: w434 -> [_ w495 w518]
                      tunnel: w433 -> [_ _ w516]
                      frame 0, Default {
                        n333 = Index Array(array=w463, index (col)=0 ("disabled index (col)")) -> (element=w465:dbl[])  [unwired: 1 in]
                        n334 = Array Size(array=w463) -> (size(s)=w469:i32[])
                        n335 = Multiply(x="after", y=25.0) -> (x*y=w467:dbl)
                        n336 = Index Array(array=w469, index=0) -> (element=w464:i32)
                        n337 = Multiply(x="before", y=25.0) -> (x*y=w468:dbl)
                        n338 = for {
                          N: w464 -> [_]
                          tunnel: w468 -> [w485]
                          tunnel: w467 -> [w487]
                          tunnel: w465 -> [w486] mode=indexing
                          shift-right: [w477] -> w462
                          shift-left: w460 -> [w481]
                          tunnel: [FALSE ("Visible")] -> w461
                          n339 = Subtract(x=w486, y=w485) -> (x-y=w483:dbl)
                          n340 = Add(x=w487, y=w486) -> (x+y=w482:dbl)
                          n341 = Array Max & Min(array=w481) -> (max value=w484:dbl, max index (indices)=w479:i32)  [unwired: 2 out]
                          n342 = Greater Or Equal?(x=w484, y=w483) -> (x >= y?=w480:bool)
                          n343 = Build Array(w483, w482) -> (w476:dbl[])
                          n344 = Build Array(w482) -> (w478:dbl[])
                          n345 = case shown="True" w480 {
                            tunnel: w481 -> [w490 w494]
                            tunnel: w479 -> [_ w493]
                            tunnel: w478 -> [_ w492]
                            tunnel: [w489 w491] -> w477
                            tunnel: w476 -> [w488 _]
                            frame False {
                              n346 = Insert Into Array(array=w490, new element=w488) -> (w489:dbl[])  [unwired: 1 in]
                            }
                            frame True {
                              n347 = Replace Array Subset(array=w494, new element=w492, index=w493) -> (w491:dbl[])
                            }
                          }
                        }
                      }
                      frame 1 {
                        n348 = for {
                          tunnel: w495 -> [w500] mode=indexing
                          shift-right: [w507] -> w497
                          shift-left: w499 -> [w508]
                          tunnel: w498 -> [w501]
                          n349 = Search 1D Array(1D array=w501, element=w500) -> (index of element=w512:i32)  [unwired: 1 in]
                          n350 = Add(x=50.0, y=w500) -> (x+y=w505:dbl)
                          n351 = Subtract(x=w512, y=1) -> (x-y=w510:i32)
                          n352 = Index Array(array=w501, index=w510) -> (element=w502:dbl)
                          n353 = Subtract(x=w502, y=50.0 ("x")) -> (x-y=w506:dbl)
                          n354 = Build Array(w506, w505) -> (w509:dbl[])
                          n355 = Insert Into Array(array=w508, new element=w509) -> (w507:dbl[])  [unwired: 1 in]
                        }
                      }
                      frame 2 {
                        n356 = Index Array(array=w516, index (col)=0 ("disabled index (col)")) -> (element=w514:dbl[])  [unwired: 1 in]
                        n357 = for {
                          tunnel: w518 -> [w522] mode=indexing
                          shift-right: [w530] -> w513
                          shift-left: w517 -> [w531]
                          tunnel: w514 -> [w525]
                          n358 = Search 1D Array(1D array=w525, element=w522) -> (index of element=w524:i32)  [unwired: 1 in]
                          n359 = Add(x=w524, y="shots") -> (x+y=w523:i32)
                          n360 = Subtract(x=w522, y=50.0 ("x")) -> (x-y=w529:dbl)
                          n361 = Index Array(array=w525, index=w523) -> (element=w521:dbl)
                          n362 = Add(x=25.0, y=w521) -> (x+y=w528:dbl)
                          n363 = Build Array(w529, w528) -> (w532:dbl[])
                          n364 = Insert Into Array(array=w531, new element=w532) -> (w530:dbl[])  [unwired: 1 in]
                        }
                      }
                    }
                  }
                }
                "edited to play" <- w341
                n365 = Index Array(array=w370, index=0) -> (element=w368:i32)
                n366 = property on="Search score" class="Slide (strict)"("Scale.Maximum"=w368, "Scale.Minimum"=0.0 ("Scale.Range:Minimum")) -> ()  [unwired: 2 in, 2 out]
                n367 = property on="Search events" class="Slide (strict)"("Visible"=w340) -> ()  [unwired: 2 in, 2 out]
                n368 = Array Size(array=w341) -> (size(s)=w363:i32)
                n369 = Divide(x=w363, y=2) -> (x/y=w359:dbl)
                n370 = for {
                  N: w359 -> [_]
                  shift-right: [w398] -> _
                  shift-left: w341 -> [w400]
                  tunnel: [w394] -> w361
                  n371 = Split 1D Array(array=w400, index=2) -> (first subarray=w399:dbl[], second subarray=w398:dbl[])
                  n372 = Index Array(array=w399, index #1=1 ("index"), index #2=0 ("index")) -> (element #1=w404:dbl, element #2=w397:dbl)
                  n373 = Subtract(x=w404, y=w397) -> (x-y=w396:dbl)
                  n374 = Increment(x=w396) -> (x+1=w395:dbl)
                  n375 = for {
                    N: w395 -> [_]
                    tunnel: w397 -> [w409]
                    tunnel: [w405] -> w394
                    i -> [w408]
                    n376 = local read "frames"() -> (w407:dbl[])
                    n377 = Add(x=w409, y=w408) -> (x+y=w406:dbl)
                    n378 = Insert Into Array(array=w407, new element=w406) -> (w405:dbl[])  [unwired: 1 in]
                    n379 = local write "frames"(w405) -> ()
                  }
                }
                n380 = local write "Playback\nscore"(w366) -> ()
                n381 = property on="Search score" class="Slide (strict)"("Visible"=w366) -> ()  [unwired: 2 in, 2 out]
                n382 = Array Size(array=w361) -> (size(s)=w358:i32)
                n383 = property on="play back" class="Slide (strict)"("Scale.Maximum"=w358, "Scale.Minimum"=w360, "Maximum"=w358) -> ()  [unwired: 2 in, 2 out]
                n384 = property on="writing" class="Slide (strict)"("Scale.Maximum"=w358, "Scale.Minimum"=w360) -> ()  [unwired: 2 in, 2 out]
                "frames" <- w362
              }
            }
            n385 = local write "edit video"(w103) -> ()
          }
          frame #1 {
            w643 = 0.0 ("X Scale.Range:Minimum")
            w682 = i16 1 ("width (-)")
            w824 = dbl[] [0.0, 0.0, 0.0, 0.0, 0.0, 0.0, 0.0, 0.0] ("array")
            w810 = string[] ["Winners", "Errors"] ("W/E1")
            w791 = string[] ["Fore hand", "Back hand", "Over head", "", "Straight", "Cross", "", "Smash", "Defence", "Drive/Tap", "Lob", "Drop", "Chop", "Clear", "Net"] ("Player 2")
            w785 = "" ("new element/subarray")
            w784 = "" ("new element/subarray")
            w737 = 9 ("index")
            w732 = 9 ("index")
            n386 = local read "edited\nevents"() -> (w703:dbl[][])
            n387 = local read "filedata in"() -> (w709:dbl[][])
            n388 = Array Size(array=w703) -> (size(s)=w715:i32[])
            n389 = Index Array(array=w709, index (col)=0 ("disabled index (col)")) -> (element=w711:dbl[])  [unwired: 1 in]
            n390 = Index Array(array=w703, index (col)=0 ("disabled index (col)")) -> (element=w708:dbl[])  [unwired: 1 in]
            n391 = Index Array(array=w715, index=0) -> (element=w713:i32)
            n392 = local read "Compare"() -> (w659:bool)
            n393 = for {
              N: w713 -> [_]
              tunnel: w711 -> [w852]
              tunnel: w708 -> [w851] mode=indexing
              tunnel: [w848] -> w701 mode=indexing
              i -> [w853]
              n394 = Search 1D Array(1D array=w852, element=w851, start index (0)=w853) -> (index of element=w849:i32)
              n395 = local read "filedata in"() -> (w850:dbl[][])
              n396 = Index Array(array=w850, index (row)=w849) -> (element=w848:dbl[])  [unwired: 1 in]
            }
            n397 = case shown="\"1\", Default" "display\nselection" {
              tunnel: [w838 w839 w840 w841] -> w702
              tunnel: w701 -> [_ w839 _ _]
              frame "1", Default {
                n398 = local read "filedata in"() -> (w838:dbl[][])
              }
              frame "2" {
              }
              frame "3" {
                n399 = local read "save1_data"() -> (w840:dbl[][])
              }
              frame "4" {
                n400 = local read "save2_data"() -> (w841:dbl[][])
              }
            }
            n401 = case shown="\"4\"" "2" {
              tunnel: [w831 w832 w833] -> w691
              frame "1", Default {
                n402 = local read "game"() -> (w831:i32[][])
              }
              frame "3" {
                n403 = local read "save1"() -> (w832:i32[][])
              }
              frame "4" {
                n404 = local read "save2"() -> (w833:i32[][])
              }
            }
            n405 = case shown="\"1\", Default" "1" {
              tunnel: [w834 w835 w836] -> w695
              frame "1", Default {
                n406 = local read "game"() -> (w834:i32[][])
              }
              frame "3" {
                n407 = local read "save1"() -> (w835:i32[][])
              }
              frame "4" {
                n408 = local read "save2"() -> (w836:i32[][])
              }
            }
            n409 = case shown="False" w659 {
              frame False {
                w825 = u8 0 ("Disabled")
                n410 = local read "Percentage"() -> (w826:bool)
                n411 = local write "Percentage"(w826) -> ()
                n412 = local read "display\nselection"() -> (w827:string)
                n413 = local write "display\nselection"(w827) -> ()
                n414 = property on="display\nselection" class="CmbBox"("Disabled"=w825) -> ()  [unwired: 2 in, 2 out]
                n415 = property on="Percentage" class="Bool (strict)"("Disabled"=w825) -> ()  [unwired: 2 in, 2 out]
              }
              frame True {
                w828 = u8 2 ("Disabled")
                n416 = local read "1"() -> (w830:string)
                n417 = local write "display\nselection"(w830) -> ()
                n418 = property on="display\nselection" class="CmbBox"("Disabled"=w828) -> ()  [unwired: 2 in, 2 out]
                n419 = property on="Percentage" class="Bool (strict)"("Disabled"=w828) -> ()  [unwired: 2 in, 2 out]
                n420 = local write "Percentage"(TRUE ("t")) -> ()
              }
            }
            n421 = Index Array(array=w691, index (row) #1=0 ("index (row)"), index (row) #2=1 ("index (row)")) -> (element #1=w689:i32[], element #2=w687:i32[])  [unwired: 2 in]
            n422 = Index Array(array=w695, index (row) #1=0 ("index (row)"), index (row) #2=1 ("index (row)")) -> (element #1=w690:i32[], element #2=w688:i32[])  [unwired: 2 in]
            n423 = Index Array(array=w702, index (col) #1=37 ("disabled index (col)"), index (col) #2=38 ("index (col)")) -> (element #1=w722:dbl[], element #2=w719:dbl[])  [unwired: 2 in]
            n424 = for {
              N: 22 -> [_]
              tunnel: w702 -> [w888]
              tunnel: w722 -> [w887]
              tunnel: w719 -> [w886]
              tunnel: [w884] -> w720 mode=indexing
              tunnel: [w883] -> w721 mode=indexing
              i -> [w881]
              n425 = Increment(x=w881) -> (x+1=w882:i32)
              n426 = Index Array(array=w888, index (col)=w882) -> (element=w885:dbl[])  [unwired: 1 in]
              n427 = And(x=w887, y=w885) -> (x .and. y?=w884:i32[])
              n428 = And(x=w886, y=w885) -> (x .and. y?=w883:i32[])
            }
            n429 = Divide(x=w690, y=w689) -> (x/y=w684:dbl[])
            n430 = Divide(x=w688, y=w687) -> (x/y=w683:dbl[])
            n431 = Index Array(array=w702, index (col) #1=23 ("disabled index (col)"), index (col) #2=25 ("index (col)"), index (col) #3=24 ("index (col)"), index (col) #4=26 ("index (col)")) -> (element #1=w793:dbl[], element #2=w798:dbl[], element #3=w799:dbl[], element #4=w797:dbl[])  [unwired: 4 in]
            n432 = Multiply(x=w683, y=100.0 ("new element/subarray")) -> (x*y=w678:dbl[])
            n433 = Multiply(x=100.0 ("new element/subarray"), y=w684) -> (x*y=w681:dbl[])
            n434 = Add Array Elements(numeric array=w793) -> (sum=w813:dbl)
            n435 = Add Array Elements(numeric array=w799) -> (sum=w812:dbl)
            n436 = local read "comp_p1 2"() -> (w657:dbl[])
            n437 = Split 1D Array(array=w681, index=22) -> (first subarray=→"comp_p1":dbl[], second subarray=→"comp_p1 2":dbl[])
            n438 = Split 1D Array(array=w678, index=22) -> (first subarray=→"comp_p2":dbl[], second subarray=→"comp_p2 2":dbl[])
            n439 = local read "Compare"() -> (w669:bool)
            n440 = local read "comp_p2 2"() -> (w665:dbl[])
            n441 = Add Array Elements(numeric array=w797) -> (sum=w811:dbl)
            n442 = Add Array Elements(numeric array=w798) -> (sum=w814:dbl)
            n443 = local read "Compare"() -> (w666:bool)
            n444 = Build Array(w813, w814) -> (w668:dbl[])
            n445 = Build Array(w812, w811) -> (w658:dbl[])
            n446 = Transpose 2D Array(2D array=w720) -> (transposed array=w731:i32[][])
            n447 = Transpose 2D Array(2D array=w721) -> (transposed array=w730:i32[][])
            n448 = Select(t=w657, s=w669, f=w668) -> (s? t:f=w667:dbl[])
            n449 = Select(t=w665, s=w666, f=w658) -> (s? t:f=w664:dbl[])
            n450 = for {
              N: 22 -> [_]
              tunnel: w731 -> [w880]
              tunnel: w730 -> [w879]
              tunnel: [w876] -> w616 mode=indexing
              tunnel: [w875] -> w604 mode=indexing
              i -> [w878]
              n451 = Index Array(array=w880, index (col)=w878) -> (element=w877:i32[])  [unwired: 1 in]
              n452 = Index Array(array=w879, index (col)=w878) -> (element=w874:i32[])  [unwired: 1 in]
              n453 = Add Array Elements(numeric array=w877) -> (sum=w876:i32)
              n454 = Add Array Elements(numeric array=w874) -> (sum=w875:i32)
            }
            n455 = Number To Decimal String(number=w667, width (-)=w682) -> (decimal integer string=→"W1/E1":string[])
            n456 = Number To Decimal String(number=w664, width (-)=w682) -> (decimal integer string=→"W2/E2":string[])
            n457 = Split 1D Array(array=w616, index=w732) -> (first subarray=w733:i32[], second subarray=w603:i32[])
            n458 = Split 1D Array(array=w604, index=w737) -> (first subarray=w736:i32[], second subarray=w741:i32[])
            n459 = Insert Into Array(array=w616, new element=w657) -> (w707:i32[])  [unwired: 1 in]
            n460 = Insert Into Array(array=w604, new element=w658) -> (w706:i32[])  [unwired: 1 in]
            n461 = Add Array Elements(numeric array=w736) -> (sum=w735:i32)
            n462 = Add Array Elements(numeric array=w733) -> (sum=w734:i32)
            n463 = Build Array(w707, w706) -> (w699:i32[][])
            n464 = Index Array(array=w741, index #1=3 ("index"), index #2=4 ("index")) -> (element #1=w729:i32, element #2=w728:i32)
            n465 = Index Array(array=w603, index #1=3 ("index"), index #2=4 ("index")) -> (element #1=w738:i32, element #2=w739:i32)
            n466 = for {
              N: w732 -> [_]
              tunnel: w733 -> [w873] mode=indexing
              tunnel: w734 -> [w872]
              tunnel: [w869] -> w762 mode=indexing
              n467 = Divide(x=w873, y=w872) -> (x/y=w871:dbl)
              n468 = Multiply(x=w871, y=100.0) -> (x*y=w869:dbl)
            }
            n469 = Add(x=w729, y=w728) -> (x+y=w740:i32)
            n470 = for {
              N: w737 -> [_]
              tunnel: w736 -> [w868] mode=indexing
              tunnel: w735 -> [w867]
              tunnel: [w864] -> w661 mode=indexing
              n471 = Divide(x=w868, y=w867) -> (x/y=w866:dbl)
              n472 = Multiply(x=w866, y=100.0) -> (x*y=w864:dbl)
            }
            n473 = Add(x=w738, y=w739) -> (x+y=w742:i32)
            n474 = case shown="\"1\"" "display\nselection" {
              tunnel: w699 -> [_ w837 _]
              frame "0", Default {
              }
              frame "1" {
                "game" <- w837
              }
              frame "2" {
              }
            }
            n475 = case shown="False" "save2" {
              tunnel: w699 -> [_ w844]
              tunnel: w702 -> [_ w842]
              frame False {
              }
              frame True {
                n476 = local write "save2"(FALSE ("save2")) -> ()
                "save2" <- w844
                "save2_data" <- w842
              }
            }
            n477 = case shown="False" "save1" {
              tunnel: w699 -> [_ w847]
              tunnel: w702 -> [_ w845]
              frame False {
              }
              frame True {
                n478 = local write "save1"(FALSE ("save1")) -> ()
                "save1" <- w847
                "save1_data" <- w845
              }
            }
            n479 = for {
              tunnel: w741 -> [w863] mode=indexing
              tunnel: w740 -> [w862]
              tunnel: [w859] -> w764 mode=indexing
              n480 = Divide(x=w863, y=w862) -> (x/y=w861:dbl)
              n481 = Multiply(x=w861, y=100.0) -> (x*y=w859:dbl)
            }
            n482 = for {
              tunnel: w603 -> [w858] mode=indexing
              tunnel: w742 -> [w857]
              tunnel: [w854] -> w763 mode=indexing
              n483 = Divide(x=w858, y=w857) -> (x/y=w856:dbl)
              n484 = Multiply(x=w856, y=100.0) -> (x*y=w854:dbl)
            }
            n485 = local read "comp_p2"() -> (w673:dbl[])
            n486 = local read "Compare"() -> (w672:bool)
            n487 = local read "comp_p1"() -> (w674:dbl[])
            n488 = Insert Into Array(array=w661, new element=w764) -> (w660:dbl[])  [unwired: 1 in]
            n489 = Insert Into Array(array=w762, new element=w763) -> (w662:dbl[])  [unwired: 1 in]
            n490 = Select(t=w673, s=w672, f=w660) -> (s? t:f=w625:dbl[])
            n491 = Select(t=w674, s="Compare", f=w662) -> (s? t:f=w620:dbl[])
            n492 = local read "Percentage"() -> (w789:bool)
            n493 = local read "Percentage"() -> (w790:bool)
            n494 = Split 1D Array(array=w625, index=9) -> (second subarray=w770:dbl[])  [unwired: 1 out]
            n495 = Number To Fractional String(number=w625, precision (6)=i16 0) -> (F-format string=w624:string[])  [unwired: 2 in]
            n496 = Split 1D Array(array=w604, index=9) -> (second subarray=w773:i32[])  [unwired: 1 out]
            n497 = Split 1D Array(array=w620, index=9) -> (second subarray=w769:dbl[])  [unwired: 1 out]
            n498 = Number To Fractional String(number=w620, precision (6)=i16 0) -> (F-format string=w617:string[])  [unwired: 2 in]
            n499 = Split 1D Array(array=w616, index=9) -> (second subarray=w767:i32[])  [unwired: 1 out]
            n500 = local read "Percentage"() -> (w777:bool)
            n501 = Number To Fractional String(number=w616, precision (6)=i16 0) -> (F-format string=w618:string[])  [unwired: 2 in]
            n502 = Number To Decimal String(number=w767, width (-)=i16 1 ("precision (6)")) -> (decimal integer string=w776:string[])
            n503 = Number To Fractional String(number=w604, precision (6)=i16 0) -> (F-format string=w622:string[])  [unwired: 2 in]
            n504 = Number To Fractional String(number=w769, precision (6)=i16 0) -> (F-format string=w775:string[])  [unwired: 2 in]
            n505 = Number To Decimal String(number=w773, width (-)=i16 1 ("precision (6)")) -> (decimal integer string=w779:string[])
            n506 = Number To Fractional String(number=w770, precision (6)=i16 0) -> (F-format string=w778:string[])  [unwired: 2 in]
            n507 = Select(t=w617, s=w790, f=w618) -> (s? t:f=w606:string[])
            n508 = Select(t=w775, s="Percentage", f=w776) -> (s? t:f=w642:string[])
            n509 = call "Search NaN_Inf (SubVI).vi"("in"=w606) -> ("out"=w605:string[])
            n510 = Select(t=w778, s=w777, f=w779) -> (s? t:f=w639:string[])
            n511 = Select(t=w624, s=w789, f=w622) -> (s? t:f=w626:string[])
            n512 = call "Search NaN_Inf (SubVI).vi"("in"=w642) -> ("out"=w641:string[])
            n513 = call "Search NaN_Inf (SubVI).vi"("in"=w626) -> ("out"=w629:string[])
            n514 = call "Search NaN_Inf (SubVI).vi"("in"=w639) -> ("out"=w640:string[])
            n515 = Insert Into Array(array=w641, index=3, new element=w784) -> (w782:string[])
            n516 = Index Array(array=w605, index #1=0 ("index"), index #2=1 ("index"), index #3=2 ("index"), index #4=3 ("index"), index #5=4 ("index"), index #6=5 ("index"), index #7=6 ("index"), index #8=7 ("index"), index #9=8 ("index")) -> (element #1=→"p1 1":string, element #2=→"p1 2":string, element #3=→"p1 3":string, element #4=→"p1 4":string, element #5=→"p1 5":string, element #6=→"p1 6":string, element #7=→"p1 7":string, element #8=→"p1 8":string, element #9=→"p1 9":string)
            n517 = Insert Into Array(array=w640, index=3, new element=w785) -> (w787:string[])
            n518 = Insert Into Array(array=w782, index=6, new element=w784) -> (w800:string[])
            n519 = Index Array(array=w629, index #1=0 ("index"), index #2=1 ("index"), index #3=2 ("index"), index #4=3 ("index"), index #5=4 ("index"), index #6=5 ("index"), index #7=6 ("index"), index #8=7 ("index"), index #9=8 ("index")) -> (element #1=→"p2 17":string, element #2=→"p2 16":string, element #3=→"p2 12":string, element #4=→"p2 13":string, element #5=→"p2 15":string, element #6=→"p2 14":string, element #7=→"p2 10":string, element #8=→"p2 11":string, element #9=→"p2 9":string)
            n520 = Insert Into Array(array=w787, index=6, new element=w785) -> (w808:string[])
            n521 = Split 1D Array(array=w800, index=6) -> (first subarray=→"player1_2":string[], second subarray=w803:string[])
            n522 = Split 1D Array(array=w808, index=6) -> (first subarray=→"player2_2":string[], second subarray=w806:string[])
            n523 = Delete From Array(array=w803, index=0) -> (array with subset deleted=w644:string[])  [unwired: 1 in, 1 out]
            "player1 2" <- w644
            n524 = Delete From Array(array=w806, index=0) -> (array with subset deleted=w645:string[])  [unwired: 1 in, 1 out]
            "player2 2" <- w645
            n525 = Fract/Exp String To Number(string=w644) -> (number=w638:dbl[])  [unwired: 3 in, 1 out]
            n526 = Fract/Exp String To Number(string=w645) -> (number=w637:dbl[])  [unwired: 3 in, 1 out]
            n527 = Array Max & Min(array=w638) -> (max value=w653:dbl)  [unwired: 3 out]
            n528 = Array Max & Min(array=w637) -> (max value=w652:dbl)  [unwired: 3 out]
            n529 = Interleave 1D Arrays(w824, w638) -> (w656:dbl[])
            n530 = Insert Into Array(array=w656, new element=0.0 ("new element/subarray")) -> (w818:dbl[])  [unwired: 1 in]
            n531 = Max & Min(x=w653, y=w652) -> (max(x,y)=w647:dbl)  [unwired: 1 out]
            n532 = Interleave 1D Arrays(w824, w637) -> (w654:dbl[])
            n533 = Bundle(w818, "array"=dbl[] [1.0, 2.0, 3.0, 4.0, 5.0, 6.0, 7.0, 8.0, 9.0, 10.0, 11.0, 12.0, 13.0, 14.0, 15.0, 16.0, 17.0]) -> (→"P1graph":cluster{dbl[], "array":dbl[]})  [unwired: 1 in]
            n534 = Equal?(x=w647, y=inf) -> (x = y?=w649:bool)
            n535 = Insert Into Array(array=w654, new element=0.0 ("new element/subarray")) -> (w819:dbl[])  [unwired: 1 in]
            n536 = Select(t=100.0, s=w649, f=w647) -> (s? t:f=w646:dbl)
            n537 = Bundle(w819, "array"=dbl[] [1.0, 2.0, 3.0, 4.0, 5.0, 6.0, 7.0, 8.0, 9.0, 10.0, 11.0, 12.0, 13.0, 14.0, 15.0, 16.0, 17.0]) -> (→"P2graph":cluster{dbl[], "array":dbl[]})  [unwired: 1 in]
            n538 = property on="P2graph" class="XYGraph (strict)"("XScale.Maximum"=w646, "XScale.Minimum"=w643) -> ()  [unwired: 2 in, 2 out]
            n539 = property on="P1graph" class="XYGraph (strict)"("XScale.Maximum"=w646, "XScale.Minimum"=w643) -> ()  [unwired: 2 in, 2 out]
            "Player 1" <- w791
            "Player 1_2" <- w791
            "Player 2_2" <- w791
            "Player 2" <- w791
            "W/E1" <- w810
            "W/E2" <- w810
          }
        }
        n540 = case shown="True" "Play" {
          frame False {
          }
          frame True {
            w948 = T5 4 items=["Grayscale (U8)", "Grayscale (I16)", "Grayscale (SGL)", "Complex (CSG)", "RGB (U32)", "HSL (U32)", "RGB (U64)"] ("Image Type")
            n541 = local read "Vid file"() -> (w936:path)
            n542 = local write "play back"(0 ("play back")) -> ()
            n543 = call "IMAQ AVI Open"("AVI Path"=w936) -> ("error out"=w939:errorcluster, "Avi Refnum"=w941:T6)  [unwired: 9 in]
            n544 = call "IMAQ Create"("Image Name"="Disp1", "Image Type"=w948) -> ("New Image"=w947:T1, "error out"=w946:errorcluster)  [unwired: 3 in]
            n545 = local write "Play"(FALSE ("Play")) -> ()
            n546 = call "IMAQ AVI Get Info"("error in (no error)"=w939, "Avi Refnum"=w941) -> ("Avi Refnum (duplicate)"=w940:T6, "Frame Data"=w938:T7)  [unwired: 5 in, 3 out]
            n547 = Unbundle By Name(w938) -> ("framesPerSecond"=w937:u32)
            n548 = while {
              tunnel: w940 -> [w968]
              tunnel: w947 -> [w970]
              tunnel: w946 -> [w969]
              tunnel: [FALSE ("Play")] -> w942
              tunnel: [w955] -> w944
              tunnel: w937 -> [w951]
              stop <- w961 stop-if-true
              n549 = local read "frames"() -> (w966:dbl[])
              n550 = Increment(x="play back") -> (x+1=w957:i32)
              n551 = Index Array(array=w966, index=w957) -> (element=w965:dbl)
              n552 = Array Max & Min(array=w966) -> (max value=w964:dbl)  [unwired: 3 out]
              n553 = Divide(x=w957, y=25.0) -> (x/y=→"Numeric":dbl)
              n554 = Divide(x=1000.0, y="Playback Speed") -> (x/y=w952:dbl)
              n555 = local write "play back"(w957) -> ()
              n556 = Divide(x=w952, y=w951) -> (x/y=w950:dbl)
              n557 = Wait (ms)(milliseconds to wait=w950) -> ()  [unwired: 1 out]
              n558 = Equal?(x=w965, y=w964) -> (x = y?=w963:bool)
              n559 = call "IMAQ AVI Read Frame"("error in (no error)"=w969, "Frame Number"=w965, "Image"=w970, "Avi Refnum"=w968) -> ("Image Out"=→"DISP":T1, "Avi Refnum (duplicate)"=w955:T6)  [unwired: 4 in, 2 out]
              n560 = Or(x=w963, y="stop 2") -> (x .or. y?=w961:bool)
              n561 = while {
                stop <- w972 continue-if-true
                n562 = local read "stop 2"() -> (w971:bool)
                n563 = Not(x=w971) -> (.not. x?=w974:bool)
                n564 = And(x=w974, y="pause") -> (x .and. y?=w972:bool)
              }
            }
            n565 = local write "stop 2"(w942) -> ()
            n566 = call "IMAQ AVI Close"("Avi Refnum"=w944) -> ()  [unwired: 10 in, 1 out]
          }
        }
        n567 = case shown="True" "write file" {
          frame False {
          }
          frame True {
            n568 = local write "writing"(0 ("writing")) -> ()
            n569 = call <vilib>:"Get File Extension.vi"("file"="Write VI") -> ("filename without extension"=w890:string)  [unwired: 7 in, 3 out]
            n570 = Strip Path(path="Write VI") -> (stripped path=w891:path)  [unwired: 1 out]
            n571 = call <vilib>:"Check if File or Folder Exists.vi"("path"=w891) -> ("file or folder exists?"=w893:bool)  [unwired: 8 in, 2 out]
            n572 = case shown="True" w893 {
              tunnel: w891 -> [_ w905]
              tunnel: w890 -> [_ w904]
              frame False {
                w895 = FALSE ("Visible")
                n573 = local write "Write VI"(path "" ("Write VI")) -> ()
                n574 = local write "write file"(w895) -> ()
                n575 = property on="writing" class="Slide (strict)"("Visible"=w895) -> ()  [unwired: 2 in, 2 out]
              }
              frame True {
                w920 = T5 4 items=["Grayscale (U8)", "Grayscale (I16)", "Grayscale (SGL)", "Complex (CSG)", "RGB (U32)", "HSL (U32)", "RGB (U64)"] ("Image Type")
                n576 = local read "Vid file"() -> (w921:path)
                n577 = Path To String(path=w905) -> (string=w907:string)
                n578 = property on="writing" class="Slide (strict)"("Visible"=TRUE) -> ()  [unwired: 2 in, 2 out]
                n579 = call "IMAQ AVI Open"("AVI Path"=w921) -> ("error out"=w901:errorcluster, "Avi Refnum"=w902:T6)  [unwired: 9 in]
                n580 = Concatenate Strings(w907, "\\" ("string"), w904, ".avi" ("string")) -> (w906:string)
                n581 = call "IMAQ AVI Get Info"("error in (no error)"=w901, "Avi Refnum"=w902) -> ("Avi Refnum (duplicate)"=w903:T6, "Frame Data"=w900:T7)  [unwired: 5 in, 3 out]
                n582 = Unbundle By Name(w900) -> ("framesPerSecond"=w899:u32)
                n583 = String To Path(string=w906) -> (path=w896:path)
                n584 = local write "Write VI"(w896) -> ()
                n585 = local read "frames"() -> (w898:dbl[])
                n586 = call "IMAQ Create"("Image Name"="write", "Image Type"=w920) -> ("New Image"=w918:T1, "error out"=w917:errorcluster)  [unwired: 3 in]
                n587 = call "IMAQ AVI Create"("Compression Filter"="Microsoft Video 1", "Frames Per Second"=w899, "AVI Path"=w896) -> ("Avi Refnum"=w922:T6)  [unwired: 7 in, 1 out]
                n588 = Array Size(array=w898) -> (size(s)=w923:i32)
                n589 = for {
                  N: w923 -> [_]
                  tunnel: w922 -> [w932]
                  tunnel: w903 -> [w925]
                  tunnel: w918 -> [w934]
                  tunnel: w917 -> [w933]
                  tunnel: [w926] -> w916
                  tunnel: [FALSE ("Play")] -> w915
                  tunnel: ["Writing complete" ("message")] -> w914
                  tunnel: [w924] -> w913
                  tunnel: [w928] -> w912
                  tunnel: w898 -> [w927] mode=indexing
                  i -> [w930]
                  n590 = call "IMAQ AVI Read Frame"("error in (no error)"=w933, "Frame Number"=w927, "Image"=w934, "Avi Refnum"=w925) -> ("error out"=w935:errorcluster, "Image Out"=w928:T1, "Avi Refnum (duplicate)"=w924:T6)  [unwired: 4 in, 1 out]
                  n591 = call "IMAQ AVI Write Frame"("error in (no error)"=w935, "Image"=w928, "Avi Refnum"=w932) -> ("Avi Refnum (duplicate)"=w926:T6)  [unwired: 7 in, 1 out]
                  "writing" <- w930
                }
                n592 = local write "write file"(w915) -> ()
                n593 = property on="writing" class="Slide (strict)"("Visible"=w915) -> ()  [unwired: 2 in, 2 out]
                n594 = call "IMAQ AVI Close"("Avi Refnum"=w916) -> ()  [unwired: 10 in, 1 out]
                n595 = call "IMAQ AVI Close"("Avi Refnum"=w913) -> ("error out"=w911:errorcluster)  [unwired: 10 in]
                n596 = One Button Dialog(message=w914) -> ()  [unwired: 1 in, 1 out]
                n597 = call "IMAQ Dispose"("Image"=w912, "error in (no error)"=w911) -> ()  [unwired: 4 in, 1 out]
              }
            }
          }
        }
        n598 = case shown="True" "REPORT" {
          frame False {
          }
          frame True {
            w102 = TRUE ("open new instance (false)")
            n599 = Automation Open(Automation Refnum="Word._Application", 9:w102) -> (Automation Refnum=w93:refnum<k7>, error out=w94:errorcluster)  [unwired: 2 in]
            n600 = Current VI's Path() -> (path=w100:path)
            n601 = property class="_Application"(reference=w93, error in=w94, "Visible"=w102) -> (reference out=w95:refnum<k7>, error out=w96:errorcluster)
            n602 = Strip Path(path=w100) -> (stripped path=w101:path)  [unwired: 1 out]
            n603 = Build Path(base path=w101, name or relative path="data\\BStAT report.doc") -> (appended path=w87:path)
            n604 = One Button Dialog(message="Right-click on the white strip on the LEFT of the data area to copy the data") -> ()  [unwired: 1 in, 1 out]
            n605 = local write "REPORT"(FALSE ("REPORT")) -> ()
            n606 = property class="_Application"(reference=w95, error in=w96) -> (error out=w98:errorcluster, "Documents"=w97:refnum<k7>)  [unwired: 1 out]
            n607 = invoke class="Documents" method="Open"(reference=w97, error in=w98, "FileName"=w87, "ReadOnly"=TRUE, "Visible"=TRUE) -> ()  [unwired: 14 in, 19 out]
          }
        }
      }
      frame True {
        w976 = u32 0 ("S_frame")
        n608 = local write "Drag control"(w976) -> ()
        n609 = local write "START"(FALSE ("START")) -> ()
        n610 = stacked-sequence {
          tunnel: w975 -> [w978 _]
          frame #0 {
            w984 = 0 ("p2code")
            w992 = T5 4 items=["Grayscale (U8)", "Grayscale (I16)", "Grayscale (SGL)", "Complex (CSG)", "RGB (U32)", "HSL (U32)", "RGB (U64)"] ("Image Type")
            n611 = call "IMAQ Create"("Image Name"="setup", "Image Type"=w992) -> ("New Image"=w990:T1, "error out"=w988:errorcluster)  [unwired: 3 in]
            n612 = call "IMAQ AVI Open"("AVI Path"=w978) -> ("Avi Refnum"=w993:T6)  [unwired: 9 in, 1 out]
            n613 = call "IMAQ AVI Get Info"("Avi Refnum"=w993) -> ("Number of Frames"=w994:u32, "Avi Refnum (duplicate)"=w986:T6, "Frame Data"=w980:T7)  [unwired: 6 in, 2 out]
            n614 = while {
              tunnel: w986 -> [w1004]
              tunnel: w990 -> [w1003]
              tunnel: w988 -> [w1002]
              tunnel: [FALSE ("Visible")] -> w981
              tunnel: [w999] -> w989
              tunnel: [w998] -> w985
              stop <- "Start Coding" stop-if-true
              w997 = TRUE ("Visible")
              n615 = while {
                tunnel: "Drag control" -> [w1010]
                stop <- w1008 stop-if-true
                n616 = local read "Drag control"() -> (w1005:u32)
                n617 = Not Equal?(x=w1010, y=w1005) -> (x != y?=w1007:bool)
                n618 = case shown="True" "F_Fr" {
                  tunnel: w1010 -> [_ w1013]
                  frame False {
                  }
                  frame True {
                    n619 = local write "F_frame"(w1013) -> ()
                    n620 = local write "F_Fr"(FALSE ("F_Fr")) -> ()
                  }
                }
                n621 = case shown="True" "S_Fr" {
                  tunnel: w1010 -> [_ w1015]
                  frame False {
                  }
                  frame True {
                    n622 = local write "S_frame"(w1015) -> ()
                    n623 = local write "S_Fr"(FALSE ("S_Fr")) -> ()
                  }
                }
                n624 = local read "Start Coding"() -> (w1006:bool)
                n625 = Or(x=w1007, y=w1006) -> (x .or. y?=w1008:bool)
              }
              n626 = call "IMAQ AVI Read Frame"("error in (no error)"=w1002, "Frame Number"="Drag control", "Image"=w1003, "Avi Refnum"=w1004) -> ("Image Out"=→"Video":T1, "Avi Refnum (duplicate)"=w999:T6)  [unwired: 4 in, 2 out]
              n627 = property on="Drag control" class="Slide (strict)"("Visible"=w997) -> ()  [unwired: 2 in, 2 out]
              n628 = property on="S_frame" class="DigNum (strict)"("Visible"=w997) -> ()  [unwired: 2 in, 2 out]
              n629 = property on="Start Coding" class="Bool (strict)"("Visible"=w997) -> ()  [unwired: 2 in, 2 out]
              n630 = property on="S_Fr" class="Bool (strict)"("Visible"=w997) -> ()  [unwired: 2 in, 2 out]
              n631 = property on="F_frame" class="DigNum (strict)"("Visible"=w997) -> ()  [unwired: 2 in, 2 out]
              n632 = property on="F_Fr" class="Bool (strict)"("Visible"=w997) -> ()  [unwired: 2 in, 2 out]
              n633 = local read "S_frame"() -> (w998:u32)
            }
            n634 = Decrement(x=w994) -> (x-1=w983:u32)
            n635 = property on="Drag control" class="Slide (strict)"("Scale.Maximum"=w983, "Scale.Minimum"=0.0 ("Scale.Range:Minimum")) -> ()  [unwired: 2 in, 2 out]
            n636 = Unbundle By Name(w980) -> ("framesPerSecond"=→"framesPerSecond":u32)
            n637 = call "IMAQ AVI Close"("Avi Refnum"=w989) -> ()  [unwired: 10 in, 1 out]
            n638 = local write "p2code"(w984) -> ()
            n639 = local write "p1code"(w984) -> ()
            n640 = local write "Start Coding"(w981) -> ()
            n641 = property on="S_frame" class="DigNum (strict)"("Visible"=w981) -> ()  [unwired: 2 in, 2 out]
            n642 = property on="F_frame" class="DigNum (strict)"("Visible"=w981) -> ()  [unwired: 2 in, 2 out]
            n643 = property on="Start Coding" class="Bool (strict)"("Visible"=w981) -> ()  [unwired: 2 in, 2 out]
            n644 = property on="S_Fr" class="Bool (strict)"("Visible"=w981) -> ()  [unwired: 2 in, 2 out]
            n645 = property on="F_Fr" class="Bool (strict)"("Visible"=w981) -> ()  [unwired: 2 in, 2 out]
            n646 = local write "Progress..."(w985) -> ()
            n647 = One Button Dialog(message="Please Select the start and end points\nof the video for coding ") -> ()  [unwired: 1 in, 1 out]
          }
          frame #1 {
            w1025 = "\r"
            w1021 = TRUE ("Visible")
            w1019 = TRUE ("Visible")
            w1040 = T5 4 items=["Grayscale (U8)", "Grayscale (I16)", "Grayscale (SGL)", "Complex (CSG)", "RGB (U32)", "HSL (U32)", "RGB (U64)"] ("Image Type")
            n648 = local read "Video file"() -> (w1029:path)
            n649 = call "IMAQ Create"("Image Name"="code", "Image Type"=w1040) -> ("New Image"=w1039:T1, "error out"=w1038:errorcluster)  [unwired: 3 in]
            n650 = call "IMAQ AVI Open"("AVI Path"=w1029) -> ("Avi Refnum"=w1037:T6)  [unwired: 9 in, 1 out]
            n651 = while {
              tunnel: w1039 -> [w1071]
              tunnel: w1038 -> [w1070]
              tunnel: w1037 -> [w1077]
              tunnel: [FALSE] -> w1022
              tunnel: [w1079] -> w1018
              tunnel: [w1076] -> w1023
              tunnel: [w1062] -> w1017
              tunnel: [w1061] -> w1016
              stop <- w1055 stop-if-true
              n652 = case shown="True" "court" {
                frame False {
                  n653 = property on="P2" class="DigNum (strict)"("Position"=T4 {"Left"=805, "Top"=395} ("Position 3")) -> ()  [unwired: 2 in, 2 out]
                  n654 = property on="P1" class="DigNum (strict)"("Position"=T4 {"Left"=805, "Top"=419} ("Position 4")) -> ()  [unwired: 2 in, 2 out]
                  n655 = property on="E2" class="Bool (strict)"("Position"=T4 {"Left"=876, "Top"=396} ("Position 28")) -> ()  [unwired: 2 in, 2 out]
                  n656 = property on="E1" class="Bool (strict)"("Position"=T4 {"Left"=876, "Top"=420} ("Position 27")) -> ()  [unwired: 2 in, 2 out]
                  n657 = property on="W1" class="Bool (strict)"("Position"=T4 {"Left"=840, "Top"=420} ("Position 19")) -> ()  [unwired: 2 in, 2 out]
                  n658 = property on="W2" class="Bool (strict)"("Position"=T4 {"Left"=840, "Top"=396} ("Position 20")) -> ()  [unwired: 2 in, 2 out]
                  n659 = property on="Pause 2" class="Bool (strict)"("Position"=T4 {"Left"=1068, "Top"=432}) -> ()  [unwired: 2 in, 2 out]
                  n660 = property on="Pause 1" class="Bool (strict)"("Position"=T4 {"Left"=1068, "Top"=456} ("Position 2")) -> ()  [unwired: 2 in, 2 out]
                  n661 = property on="TL 3" class="Bool (strict)"("Position"=T4 {"Left"=804, "Top"=235} ("Position 5")) -> ()  [unwired: 2 in, 2 out]
                  n662 = property on="TL 2" class="Bool (strict)"("Position"=T4 {"Left"=876, "Top"=204} ("Position 6")) -> ()  [unwired: 2 in, 2 out]
                  n663 = property on="CL 3" class="Bool (strict)"("Position"=T4 {"Left"=804, "Top"=259} ("Position 7")) -> ()  [unwired: 2 in, 2 out]
                  n664 = property on="CL 2" class="Bool (strict)"("Position"=T4 {"Left"=876, "Top"=180} ("Position 8")) -> ()  [unwired: 2 in, 2 out]
                  n665 = property on="BL 3" class="Bool (strict)"("Position"=T4 {"Left"=804, "Top"=283} ("Position 9")) -> ()  [unwired: 2 in, 2 out]
                  n666 = property on="BL 2" class="Bool (strict)"("Position"=T4 {"Left"=876, "Top"=156} ("Position 10")) -> ()  [unwired: 2 in, 2 out]
                  n667 = property on="S1" class="Bool (strict)"("Position"=T4 {"Left"=936, "Top"=432} ("Position 11")) -> ()  [unwired: 2 in, 2 out]
                  n668 = property on="S2" class="Bool (strict)"("Position"=T4 {"Left"=936, "Top"=384} ("Position 12")) -> ()  [unwired: 2 in, 2 out]
                  n669 = property on="TM 3" class="Bool (strict)"("Position"=T4 {"Left"=840, "Top"=235} ("Position 13")) -> ()  [unwired: 2 in, 2 out]
                  n670 = property on="TM 2" class="Bool (strict)"("Position"=T4 {"Left"=840, "Top"=204} ("Position 14")) -> ()  [unwired: 2 in, 2 out]
                  n671 = property on="CM 3" class="Bool (strict)"("Position"=T4 {"Left"=840, "Top"=259} ("Position 15")) -> ()  [unwired: 2 in, 2 out]
                  n672 = property on="CM 2" class="Bool (strict)"("Position"=T4 {"Left"=840, "Top"=180} ("Position 16")) -> ()  [unwired: 2 in, 2 out]
                  n673 = property on="BM 3" class="Bool (strict)"("Position"=T4 {"Left"=840, "Top"=283} ("Position 17")) -> ()  [unwired: 2 in, 2 out]
                  n674 = property on="BM 2" class="Bool (strict)"("Position"=T4 {"Left"=840, "Top"=156} ("Position 18")) -> ()  [unwired: 2 in, 2 out]
                  n675 = property on="TR 3" class="Bool (strict)"("Position"=T4 {"Left"=876, "Top"=235} ("Position 21")) -> ()  [unwired: 2 in, 2 out]
                  n676 = property on="TR 2" class="Bool (strict)"("Position"=T4 {"Left"=804, "Top"=204} ("Position 22")) -> ()  [unwired: 2 in, 2 out]
                  n677 = property on="CR  3" class="Bool (strict)"("Position"=T4 {"Left"=876, "Top"=259} ("Position 23")) -> ()  [unwired: 2 in, 2 out]
                  n678 = property on="CR  2" class="Bool (strict)"("Position"=T4 {"Left"=804, "Top"=180} ("Position 24")) -> ()  [unwired: 2 in, 2 out]
                  n679 = property on="BR 3" class="Bool (strict)"("Position"=T4 {"Left"=876, "Top"=283} ("Position 25")) -> ()  [unwired: 2 in, 2 out]
                  n680 = property on="BR 2" class="Bool (strict)"("Position"=T4 {"Left"=804, "Top"=156} ("Position 26")) -> ()  [unwired: 2 in, 2 out]
                }
                frame True {
                  n681 = property on="P2" class="DigNum (strict)"("Position"=T4 {"Left"=805, "Top"=419} ("Position 3")) -> ()  [unwired: 2 in, 2 out]
                  n682 = property on="P1" class="DigNum (strict)"("Position"=T4 {"Left"=805, "Top"=395} ("Position 4")) -> ()  [unwired: 2 in, 2 out]
                  n683 = property on="E2" class="Bool (strict)"("Position"=T4 {"Left"=876, "Top"=420} ("Position 28")) -> ()  [unwired: 2 in, 2 out]
                  n684 = property on="E1" class="Bool (strict)"("Position"=T4 {"Left"=876, "Top"=396} ("Position 27")) -> ()  [unwired: 2 in, 2 out]
                  n685 = property on="W1" class="Bool (strict)"("Position"=T4 {"Left"=840, "Top"=396} ("Position 19")) -> ()  [unwired: 2 in, 2 out]
                  n686 = property on="W2" class="Bool (strict)"("Position"=T4 {"Left"=840, "Top"=420} ("Position 20")) -> ()  [unwired: 2 in, 2 out]
                  n687 = property on="Pause 2" class="Bool (strict)"("Position"=T4 {"Left"=1068, "Top"=456}) -> ()  [unwired: 2 in, 2 out]
                  n688 = property on="Pause 1" class="Bool (strict)"("Position"=T4 {"Left"=1068, "Top"=432} ("Position 2")) -> ()  [unwired: 2 in, 2 out]
                  n689 = property on="TL 3" class="Bool (strict)"("Position"=T4 {"Left"=876, "Top"=204} ("Position 6")) -> ()  [unwired: 2 in, 2 out]
                  n690 = property on="TL 2" class="Bool (strict)"("Position"=T4 {"Left"=804, "Top"=235} ("Position 5")) -> ()  [unwired: 2 in, 2 out]
                  n691 = property on="CL 3" class="Bool (strict)"("Position"=T4 {"Left"=876, "Top"=180} ("Position 8")) -> ()  [unwired: 2 in, 2 out]
                  n692 = property on="CL 2" class="Bool (strict)"("Position"=T4 {"Left"=804, "Top"=259} ("Position 7")) -> ()  [unwired: 2 in, 2 out]
                  n693 = property on="BL 3" class="Bool (strict)"("Position"=T4 {"Left"=876, "Top"=156} ("Position 10")) -> ()  [unwired: 2 in, 2 out]
                  n694 = property on="BL 2" class="Bool (strict)"("Position"=T4 {"Left"=804, "Top"=283} ("Position 9")) -> ()  [unwired: 2 in, 2 out]
                  n695 = property on="S1" class="Bool (strict)"("Position"=T4 {"Left"=936, "Top"=384} ("Position 11")) -> ()  [unwired: 2 in, 2 out]
                  n696 = property on="S2" class="Bool (strict)"("Position"=T4 {"Left"=936, "Top"=432} ("Position 12")) -> ()  [unwired: 2 in, 2 out]
                  n697 = property on="TM 3" class="Bool (strict)"("Position"=T4 {"Left"=840, "Top"=204} ("Position 14")) -> ()  [unwired: 2 in, 2 out]
                  n698 = property on="TM 2" class="Bool (strict)"("Position"=T4 {"Left"=840, "Top"=235} ("Position 13")) -> ()  [unwired: 2 in, 2 out]
                  n699 = property on="CM 3" class="Bool (strict)"("Position"=T4 {"Left"=840, "Top"=180} ("Position 16")) -> ()  [unwired: 2 in, 2 out]
                  n700 = property on="CM 2" class="Bool (strict)"("Position"=T4 {"Left"=840, "Top"=259} ("Position 15")) -> ()  [unwired: 2 in, 2 out]
                  n701 = property on="BM 3" class="Bool (strict)"("Position"=T4 {"Left"=840, "Top"=156} ("Position 18")) -> ()  [unwired: 2 in, 2 out]
                  n702 = property on="BM 2" class="Bool (strict)"("Position"=T4 {"Left"=840, "Top"=283} ("Position 17")) -> ()  [unwired: 2 in, 2 out]
                  n703 = property on="TR 3" class="Bool (strict)"("Position"=T4 {"Left"=804, "Top"=204} ("Position 22")) -> ()  [unwired: 2 in, 2 out]
                  n704 = property on="TR 2" class="Bool (strict)"("Position"=T4 {"Left"=876, "Top"=235} ("Position 21")) -> ()  [unwired: 2 in, 2 out]
                  n705 = property on="CR  3" class="Bool (strict)"("Position"=T4 {"Left"=804, "Top"=180} ("Position 24")) -> ()  [unwired: 2 in, 2 out]
                  n706 = property on="CR  2" class="Bool (strict)"("Position"=T4 {"Left"=876, "Top"=259} ("Position 23")) -> ()  [unwired: 2 in, 2 out]
                  n707 = property on="BR 3" class="Bool (strict)"("Position"=T4 {"Left"=804, "Top"=156} ("Position 26")) -> ()  [unwired: 2 in, 2 out]
                  n708 = property on="BR 2" class="Bool (strict)"("Position"=T4 {"Left"=876, "Top"=283} ("Position 25")) -> ()  [unwired: 2 in, 2 out]
                }
              }
              n709 = Increment(x="Progress...") -> (x+1=w1078:i32)
              n710 = call "IMAQ AVI Read Frame"("error in (no error)"=w1070, "Frame Number"=w1078, "Image"=w1071, "Avi Refnum"=w1077) -> ("Image Out"=w1054:T1)  [unwired: 4 in, 3 out]
              n711 = local write "Video"(w1054) -> ()
              n712 = local read "F_frame"() -> (w1082:u32)
              n713 = Add(x=9, y=w1078) -> (x+y=w1081:i32)
              n714 = Less Or Equal?(x=w1082, y=w1081) -> (x <= y?=w1059:bool)
              n715 = local read "framesPerSecond"() -> (w1053:u32)
              n716 = Select(t=w1081, s="fast forward", f=w1078) -> (s? t:f=w1058:i32)
              n717 = Select(t="Progress...", s=w1059, f=w1058) -> (s? t:f=w1056:i32)
              n718 = Divide(x=1000.0, y="playback speed") -> (x/y=w1085:dbl)
              n719 = local write "Progress..."(w1056) -> ()
              n720 = Divide(x=w1085, y=w1053) -> (x/y=w1052:dbl)
              n721 = Wait (ms)(milliseconds to wait=w1052) -> ()  [unwired: 1 out]
              n722 = Compound Arithmetic op=OR("Pause 1", "Pause 2", "Pause 3") -> (w1080:bool)
              n723 = case shown="True" w1080 {
                tunnel: w1078 -> [w1161 w1241]
                tunnel: [w1160 w1226] -> w1079
                tunnel: w1078 -> [_ w1244]
                tunnel: w1077 -> [w1158 w1243]
                tunnel: [w1158 w1240] -> w1076
                tunnel: "Pause 1" -> [_ w1239]
                tunnel: "Pause 2" -> [_ w1238]
                tunnel: w1052 -> [_ w1234]
                frame False {
                  n724 = local read "W1"() -> (w1157:bool)
                  n725 = local read "W2"() -> (w1155:bool)
                  n726 = local read "E1"() -> (w1156:bool)
                  n727 = local read "E2"() -> (w1154:bool)
                  n728 = Or(x=w1157, y=w1156) -> (x .or. y?=w1153:bool)
                  n729 = Or(x=w1155, y=w1154) -> (x .or. y?=w1152:bool)
                  n730 = Boolean To (0,1)(Boolean=w1153) -> (0, 1=w1150:i16)
                  n731 = Select(t=2.0, s=w1152, f=w1150) -> (s? t:f=w1149:dbl)
                  n732 = case shown="0, Default" w1149 {
                    tunnel: w1161 -> [_ _ _]
                    tunnel: [w1164 w1193 w1196] -> w1160
                    tunnel: [FALSE FALSE FALSE] -> w1159
                    frame 0, Default {
                      w1162 = FALSE ("4 6")
                      n733 = local write "1 6"(w1162) -> ()
                      n734 = local write "2 6"(w1162) -> ()
                      n735 = local write "3 6"(w1162) -> ()
                      n736 = local write "4 6"(w1162) -> ()
                      n737 = local write "5 6"(w1162) -> ()
                      n738 = local write "6 6"(w1162) -> ()
                      n739 = local write "7 6"(w1162) -> ()
                      n740 = local write "8 6"(w1162) -> ()
                      n741 = local write "1 5"(w1162) -> ()
                      n742 = local write "2 5"(w1162) -> ()
                      n743 = local write "3 5"(w1162) -> ()
                      n744 = local write "4 5"(w1162) -> ()
                      n745 = local write "5 5"(w1162) -> ()
                      n746 = local write "6 5"(w1162) -> ()
                      n747 = local write "7 5"(w1162) -> ()
                      n748 = local write "8 5"(w1162) -> ()
                      n749 = local write "1 4"(w1162) -> ()
                      n750 = local write "2 4"(w1162) -> ()
                      n751 = local write "3 4"(w1162) -> ()
                      n752 = local write "4 4"(w1162) -> ()
                      n753 = local write "5 4"(w1162) -> ()
                      n754 = local write "6 4"(w1162) -> ()
                      n755 = local write "7 4"(w1162) -> ()
                      n756 = local write "8 4"(w1162) -> ()
                      n757 = local write "1 3"(w1162) -> ()
                      n758 = local write "2 3"(w1162) -> ()
                      n759 = local write "3 3"(w1162) -> ()
                      n760 = local write "4 3"(w1162) -> ()
                      n761 = local write "5 3"(w1162) -> ()
                      n762 = local write "6 3"(w1162) -> ()
                      n763 = local write "7 3"(w1162) -> ()
                      n764 = local write "8 3"(w1162) -> ()
                      n765 = local write "1 2"(w1162) -> ()
                      n766 = local write "2 2"(w1162) -> ()
                      n767 = local write "3 2"(w1162) -> ()
                      n768 = local write "4 2"(w1162) -> ()
                      n769 = local write "5 2"(w1162) -> ()
                      n770 = local write "6 2"(w1162) -> ()
                      n771 = local write "7 2"(w1162) -> ()
                      n772 = local write "8 2"(w1162) -> ()
                      n773 = local write "1"(w1162) -> ()
                      n774 = local write "2"(w1162) -> ()
                      n775 = local write "3"(w1162) -> ()
                      n776 = local write "4"(w1162) -> ()
                      n777 = local write "5"(w1162) -> ()
                      n778 = local write "6"(w1162) -> ()
                      n779 = local write "7"(w1162) -> ()
                      n780 = local write "8"(w1162) -> ()
                      n781 = local write "BL 3"(w1162) -> ()
                      n782 = local write "BL 2"(w1162) -> ()
                      n783 = local write "BM 3"(w1162) -> ()
                      n784 = local write "BM 2"(w1162) -> ()
                      n785 = local write "BR 2"(w1162) -> ()
                      n786 = local write "BR 3"(w1162) -> ()
                      n787 = local write "W1"(w1162) -> ()
                      n788 = local write "W2"(w1162) -> ()
                      n789 = local write "E1"(w1162) -> ()
                      n790 = local write "E2"(w1162) -> ()
                      n791 = local write "TL 3"(w1162) -> ()
                      n792 = local write "TL 2"(w1162) -> ()
                      n793 = local write "TM 2"(w1162) -> ()
                      n794 = local write "TM 3"(w1162) -> ()
                      n795 = local write "TR 2"(w1162) -> ()
                      n796 = local write "TR 3"(w1162) -> ()
                      n797 = local write "S1"(w1162) -> ()
                      n798 = local write "S2"(w1162) -> ()
                      n799 = local write "1"(w1162) -> ()
                      n800 = local write "2"(w1162) -> ()
                      n801 = local write "3"(w1162) -> ()
                      n802 = local write "4"(w1162) -> ()
                      n803 = local write "CL 3"(w1162) -> ()
                      n804 = local write "CL 2"(w1162) -> ()
                      n805 = local write "CM 2"(w1162) -> ()
                      n806 = local write "CM 3"(w1162) -> ()
                      n807 = local write "CR  2"(w1162) -> ()
                      n808 = local write "CR  3"(w1162) -> ()
                      n809 = local read "coding"() -> (w1164:i32[][])
                    }
                    frame 1 {
                      n810 = local read "W1"() -> (w1187:bool)
                      n811 = local read "W2"() -> (w1188:bool)
                      n812 = local read "E1"() -> (w1189:bool)
                      n813 = local read "E2"() -> (w1190:bool)
                      n814 = Boolean To (0,1)(Boolean=w1187) -> (0, 1=w1179:i16)
                      n815 = Boolean To (0,1)(Boolean=w1188) -> (0, 1=w1178:i16)
                      n816 = Boolean To (0,1)(Boolean=w1189) -> (0, 1=w1173:i16)
                      n817 = Boolean To (0,1)(Boolean=w1190) -> (0, 1=w1172:i16)
                      n818 = Or(x=w1187, y=w1190) -> (x .or. y?=w1186:bool)
                      n819 = Or(x=w1188, y=w1189) -> (x .or. y?=w1185:bool)
                      n820 = local read "P2"() -> (w1165:i32)
                      n821 = local read "P1"() -> (w1191:i32)
                      n822 = Increment(x=w1191) -> (x+1=w1184:i32)
                      n823 = Increment(x=w1165) -> (x+1=w1183:i32)
                      n824 = Select(t=w1183, s=w1185, f=w1165) -> (s? t:f=w1166:i32)
                      n825 = Select(t=w1184, s=w1186, f=w1191) -> (s? t:f=w1168:i32)
                      n826 = Boolean To (0,1)(Boolean=w1186) -> (0, 1=w1171:i16)
                      n827 = Boolean To (0,1)(Boolean=w1185) -> (0, 1=w1170:i16)
                      n828 = local write "P1"(w1168) -> ()
                      n829 = local write "P2"(w1166) -> ()
                      n830 = local read "p1code"() -> (w1181:i32)
                      n831 = local read "coding"() -> (w1192:i32[][])
                      n832 = Replace Array Subset(array=w1192, new element #1=w1179, index (row) #1=w1181, index (col) #1=23 ("disabled index (col)"), new element #2=w1178, index (row) #2=w1181, index (col) #2=24 ("disabled index (col)"), new element #3=w1173, index (row) #3=w1181, index (col) #3=25 ("disabled index (col)"), new element #4=w1172, index (row) #4=w1181, index (col) #4=26 ("disabled index (col)"), new element #5=w1171, index (row) #5=w1181, index (col) #5=27 ("disabled index (col)"), new element #6=w1170, index (row) #6=w1181, index (col) #6=28 ("disabled index (col)"), new element #7=w1168, index (row) #7=w1181, index (col) #7=29 ("disabled index (col)"), new element #8=w1166, index (row) #8=w1181, index (col) #8=30 ("disabled index (col)")) -> (w1193:i32[][])
                      n833 = local write "coding"(w1193) -> ()
                    }
                    frame 2 {
                      n834 = local read "W1"() -> (w1219:bool)
                      n835 = local read "W2"() -> (w1220:bool)
                      n836 = local read "E1"() -> (w1221:bool)
                      n837 = local read "E2"() -> (w1222:bool)
                      n838 = Boolean To (0,1)(Boolean=w1219) -> (0, 1=w1212:i16)
                      n839 = Boolean To (0,1)(Boolean=w1220) -> (0, 1=w1211:i16)
                      n840 = Boolean To (0,1)(Boolean=w1221) -> (0, 1=w1206:i16)
                      n841 = Boolean To (0,1)(Boolean=w1222) -> (0, 1=w1205:i16)
                      n842 = Or(x=w1219, y=w1222) -> (x .or. y?=w1218:bool)
                      n843 = Or(x=w1220, y=w1221) -> (x .or. y?=w1217:bool)
                      n844 = local read "P2"() -> (w1195:i32)
                      n845 = local read "P1"() -> (w1223:i32)
                      n846 = Increment(x=w1223) -> (x+1=w1216:i32)
                      n847 = Increment(x=w1195) -> (x+1=w1215:i32)
                      n848 = Select(t=w1215, s=w1217, f=w1195) -> (s? t:f=w1199:i32)
                      n849 = Select(t=w1216, s=w1218, f=w1223) -> (s? t:f=w1201:i32)
                      n850 = Boolean To (0,1)(Boolean=w1218) -> (0, 1=w1204:i16)
                      n851 = Boolean To (0,1)(Boolean=w1217) -> (0, 1=w1203:i16)
                      n852 = local write "P1"(w1201) -> ()
                      n853 = local write "P2"(w1199) -> ()
                      n854 = local read "p2code"() -> (w1197:i32)
                      n855 = local read "coding"() -> (w1224:i32[][])
                      n856 = Replace Array Subset(array=w1224, new element #1=w1212, index (row) #1=w1197, index (col) #1=23 ("disabled index (col)"), new element #2=w1211, index (row) #2=w1197, index (col) #2=24 ("disabled index (col)"), new element #3=w1206, index (row) #3=w1197, index (col) #3=25 ("disabled index (col)"), new element #4=w1205, index (row) #4=w1197, index (col) #4=26 ("disabled index (col)"), new element #5=w1204, index (row) #5=w1197, index (col) #5=27 ("disabled index (col)"), new element #6=w1203, index (row) #6=w1197, index (col) #6=28 ("disabled index (col)"), new element #7=w1201, index (row) #7=w1197, index (col) #7=29 ("disabled index (col)"), new element #8=w1199, index (row) #8=w1197, index (col) #8=30 ("disabled index (col)")) -> (w1196:i32[][])
                      n857 = local write "coding"(w1196) -> ()
                    }
                  }
                  n858 = local write "W1"(w1159) -> ()
                  n859 = local write "W2"(w1159) -> ()
                  n860 = local write "E1"(w1159) -> ()
                  n861 = local write "E2"(w1159) -> ()
                }
                frame True {
                  n862 = stacked-sequence {
                    tunnel: [_ w1327 _ _ _ _ _ _] -> w1242
                    tunnel: [_ w1326 _ _ _ _ _ _] -> w1281
                    tunnel: [_ w1325 _ _ _ _ _ _] -> w1280
                    tunnel: [_ w1324 _ _ _ _ _ _] -> w1279
                    tunnel: [_ w1323 _ _ _ _ _ _] -> w1278
                    tunnel: [_ w1322 _ _ _ _ _ _] -> w1277
                    tunnel: [_ w1321 _ _ _ _ _ _] -> w1276
                    tunnel: [_ w1320 _ _ _ _ _ _] -> w1270
                    tunnel: [_ w1319 _ _ _ _ _ _] -> w1275
                    tunnel: [_ _ _ w1397 _ _ _ _] -> w1274
                    tunnel: [_ _ _ w1396 _ _ _ _] -> w1273
                    tunnel: [_ _ _ w1394 _ _ _ _] -> w1272
                    tunnel: [_ _ _ _ w1494 _ _ _] -> w1271
                    tunnel: [_ _ _ _ w1491 _ _ _] -> w1269
                    tunnel: [_ _ _ _ w1458 _ _ _] -> w1268
                    tunnel: [_ _ _ _ w1457 _ _ _] -> w1267
                    tunnel: [_ _ _ _ w1456 _ _ _] -> w1266
                    tunnel: [_ _ _ _ w1455 _ _ _] -> w1265
                    tunnel: [_ _ _ _ w1454 _ _ _] -> w1264
                    tunnel: [_ _ _ _ w1453 _ _ _] -> w1263
                    tunnel: [_ _ _ _ w1452 _ _ _] -> w1262
                    tunnel: [_ _ _ _ w1451 _ _ _] -> w1261
                    tunnel: [_ _ _ _ _ _ w1579 _] -> w1260
                    tunnel: [_ _ _ _ _ _ w1579 _] -> w1259
                    tunnel: [_ _ _ _ _ _ w1579 _] -> w1258
                    tunnel: [_ _ _ _ _ _ w1579 _] -> w1257
                    tunnel: [_ _ _ _ _ _ w1579 _] -> w1256
                    tunnel: [_ _ _ _ _ _ w1579 _] -> w1255
                    tunnel: [_ _ _ _ _ _ w1579 _] -> w1254
                    tunnel: [_ _ _ _ _ _ w1579 _] -> w1253
                    tunnel: [_ _ _ _ _ _ w1585 _] -> w1252
                    tunnel: [_ _ _ _ _ _ w1584 _] -> w1251
                    tunnel: [_ _ _ _ _ _ w1583 _] -> w1250
                    tunnel: [_ _ _ _ _ _ w1582 _] -> w1249
                    tunnel: [_ _ _ _ _ _ w1581 _] -> w1248
                    tunnel: [_ _ _ _ _ _ w1580 _] -> w1247
                    tunnel: [_ _ w1365 _ _ _ _ _] -> w1246
                    tunnel: [_ _ w1364 _ _ _ _ _] -> w1245
                    tunnel: w1244 -> [w1290 _ _ _ _ _ _ _]
                    tunnel: w1243 -> [w1289 _ _ _ _ _ _ _]
                    tunnel: [w1288 _ _ _ _ _ _ _] -> w1240
                    tunnel: [_ _ _ _ _ _ _ w1592] -> w1227
                    tunnel: w1239 -> [_ _ w1363 _ _ _ _ _]
                    tunnel: w1238 -> [_ _ w1362 _ _ _ _ _]
                    tunnel: w1234 -> [w1283 _ _ _ _ _ _ _]
                    tunnel: [w1282 _ _ _ _ _ _ _] -> w1225
                    frame #0 {
                      w1286 = T5 4 items=["Grayscale (U8)", "Grayscale (I16)", "Grayscale (SGL)", "Complex (CSG)", "RGB (U32)", "HSL (U32)", "RGB (U64)"] ("Image Type")
                      n863 = while {
                        tunnel: [FALSE] -> w1287
                        stop <- w1312 continue-if-true
                        n864 = local read "Pause 3"() -> (w1309:bool)
                        n865 = local read "Pause 1"() -> (w1310:bool)
                        n866 = local read "Pause 2"() -> (w1313:bool)
                        n867 = local read "coding"() -> (w1304:i32[][])
                        n868 = Compound Arithmetic op=OR(w1309, w1310, w1313) -> (w1312:bool)
                        n869 = Index Array(array=w1304, index (col)=0 ("disabled index (col)")) -> (element=w1307:i32[])  [unwired: 1 in]
                        n870 = Array Max & Min(array=w1307) -> (max value=w1306:i32, max index (indices)=w1303:i32)  [unwired: 2 out]
                        n871 = call "Time Delay4"("Delay Time (s)"=0.01) -> ()  [unwired: 10 in, 1 out]
                        n872 = case shown="True" "UNDO" {
                          selector: "UNDO" -> [w1314 _]
                          tunnel: w1304 -> [_ w1318]
                          tunnel: w1303 -> [_ w1317]
                          tunnel: [w1314 FALSE] -> w1302
                          frame False {
                          }
                          frame True {
                            n873 = Delete From Array(array=w1318, index (row)=w1317) -> (array with subset deleted=w1316:i32[][])  [unwired: 2 in, 1 out]
                            n874 = local write "coding"(w1316) -> ()
                          }
                        }
                        n875 = local write "Last coded"(w1306) -> ()
                        n876 = local write "UNDO"(w1302) -> ()
                      }
                      n877 = call "IMAQ Create"("Image Name"="code3", "Image Type"=w1286) -> ("New Image"=w1282:T1, "error out"=w1284:errorcluster)  [unwired: 3 in]
                      n878 = for {
                        N: 25 -> [_]
                        tunnel: w1290 -> [w1299]
                        tunnel: w1289 -> [w1297]
                        tunnel: w1284 -> [w1296]
                        tunnel: w1282 -> [w1295]
                        tunnel: [w1294] -> w1288
                        tunnel: w1283 -> [w1293]
                        i -> [w1300]
                        n879 = Add(x=w1300, y=w1299) -> (x+y=w1298:i32)
                        n880 = call "IMAQ AVI Read Frame"("error in (no error)"=w1296, "Frame Number"=w1298, "Image"=w1295, "Avi Refnum"=w1297) -> ("Image Out"=w1292:T1, "Avi Refnum (duplicate)"=w1294:T6)  [unwired: 4 in, 2 out]
                        n881 = local write "Video"(w1292) -> ()
                        n882 = Wait (ms)(milliseconds to wait=w1293) -> ()  [unwired: 1 out]
                      }
                      n883 = local write "Pause 1"(w1287) -> ()
                      n884 = local write "Pause 2"(w1287) -> ()
                      n885 = local write "Pause 3"(w1287) -> ()
                      n886 = local write "UNDO"(w1287) -> ()
                    }
                    frame #1 {
                      n887 = Or(x="TM 2", y="TM 3") -> (x .or. y?=w1335:bool)
                      n888 = Or(x="CL 3", y="CL 2") -> (x .or. y?=w1333:bool)
                      n889 = Or(x="CR  2", y="CR  3") -> (x .or. y?=w1331:bool)
                      n890 = Or(x="BM 3", y="BM 2") -> (x .or. y?=w1329:bool)
                      n891 = Boolean To (0,1)(Boolean=w1335) -> (0, 1=w1326:i16)
                      n892 = Boolean To (0,1)(Boolean=w1333) -> (0, 1=w1324:i16)
                      n893 = Boolean To (0,1)(Boolean=w1331) -> (0, 1=w1322:i16)
                      n894 = Boolean To (0,1)(Boolean=w1329) -> (0, 1=w1320:i16)
                      n895 = Or(x="TL 3", y="TL 2") -> (x .or. y?=w1336:bool)
                      n896 = Or(x="TR 2", y="TR 3") -> (x .or. y?=w1334:bool)
                      n897 = Or(x="CM 2", y="CM 3") -> (x .or. y?=w1332:bool)
                      n898 = Or(x="BL 3", y="BL 2") -> (x .or. y?=w1330:bool)
                      n899 = Or(x="BR 2", y="BR 3") -> (x .or. y?=w1328:bool)
                      n900 = Boolean To (0,1)(Boolean=w1336) -> (0, 1=w1327:i16)
                      n901 = Boolean To (0,1)(Boolean=w1334) -> (0, 1=w1325:i16)
                      n902 = Boolean To (0,1)(Boolean=w1332) -> (0, 1=w1323:i16)
                      n903 = Boolean To (0,1)(Boolean=w1330) -> (0, 1=w1321:i16)
                      n904 = Boolean To (0,1)(Boolean=w1328) -> (0, 1=w1319:i16)
                    }
                    frame #2 {
                      n905 = local read "S1"() -> (w1361:bool)
                      n906 = local read "S2"() -> (w1360:bool)
                      n907 = local read "CM 3"() -> (w1389:bool)
                      n908 = local read "TM 3"() -> (w1390:bool)
                      n909 = local read "BM 3"() -> (w1388:bool)
                      n910 = local read "CR  3"() -> (w1385:bool)
                      n911 = local read "CL 3"() -> (w1391:bool)
                      n912 = local read "BR 3"() -> (w1387:bool)
                      n913 = local read "TR 3"() -> (w1386:bool)
                      n914 = local read "BL 3"() -> (w1393:bool)
                      n915 = local read "TL 3"() -> (w1392:bool)
                      n916 = Or(x=w1361, y=w1360) -> (x .or. y?=w1356:bool)
                      n917 = Compound Arithmetic op=OR(w1393, w1392, w1391, w1390, w1389, w1388, w1387, w1386, w1385) -> (w1367:bool)
                      "P1 position" <- w1367
                      n918 = Or(x=w1367, y=w1363) -> (x .or. y?=w1358:bool)
                      n919 = Or(x=w1358, y=w1356) -> (x .or. y?=w1359:bool)
                      n920 = local read "coding"() -> (w1375:i32[][])
                      n921 = local read "CM 2"() -> (w1381:bool)
                      n922 = local read "TM 2"() -> (w1382:bool)
                      n923 = local read "BM 2"() -> (w1380:bool)
                      n924 = local read "CR  2"() -> (w1379:bool)
                      n925 = local read "CL 2"() -> (w1376:bool)
                      n926 = local read "TR 2"() -> (w1378:bool)
                      n927 = local read "BR 2"() -> (w1377:bool)
                      n928 = local read "BL 2"() -> (w1384:bool)
                      n929 = local read "TL 2"() -> (w1383:bool)
                      n930 = Boolean To (0,1)(Boolean=w1359) -> (0, 1=w1365:i16)
                      n931 = Array Size(array=w1375) -> (size(s)=w1374:i32[])
                      n932 = Compound Arithmetic op=OR(w1384, w1383, w1376, w1382, w1381, w1380, w1379, w1378, w1377) -> (w1366:bool)
                      "P2 position" <- w1366
                      n933 = local read "p1code"() -> (w1371:i32)
                      n934 = Index Array(array=w1374, index=0) -> (element=w1369:i32)
                      n935 = Or(x=w1366, y=w1362) -> (x .or. y?=w1357:bool)
                      n936 = Or(x=w1357, y=w1356) -> (x .or. y?=w1355:bool)
                      n937 = Select(t=w1369, s=w1359, f=w1371) -> (s? t:f=→"p1code":i32)
                      n938 = local read "p2code"() -> (w1368:i32)
                      n939 = Select(t=w1369, s=w1355, f=w1368) -> (s? t:f=→"p2code":i32)
                      n940 = Boolean To (0,1)(Boolean=w1355) -> (0, 1=w1364:i16)
                    }
                    frame #3 {
                      n941 = Build Array("1", "2", "3", "4", "5", "6", "7", "8", "1 2", "2 2", "3 2", "4 2", "5 2", "6 2", "7 2", "8 2") -> (w1418:bool[])
                      "FH" <- w1418
                      n942 = Or Array Elements(Boolean array=w1418) -> (logical OR=w1399:bool)
                      n943 = Boolean To (0,1)(Boolean=w1399) -> (0, 1=w1397:i16)
                      n944 = Build Array("1 3", "2 3", "3 3", "4 3", "5 3", "6 3", "7 3", "8 3", "1 4", "2 4", "3 4", "4 4", "5 4", "6 4", "7 4", "8 4") -> (w1401:bool[])
                      "BH" <- w1401
                      n945 = Or Array Elements(Boolean array=w1401) -> (logical OR=w1398:bool)
                      n946 = Boolean To (0,1)(Boolean=w1398) -> (0, 1=w1396:i16)
                      n947 = Build Array("1 5", "2 5", "3 5", "4 5", "5 5", "6 5", "7 5", "8 5", "1 6", "2 6", "3 6", "4 6", "5 6", "6 6", "7 6", "8 6") -> (w1400:bool[])
                      "OH" <- w1400
                      n948 = Or Array Elements(Boolean array=w1400) -> (logical OR=w1395:bool)
                      n949 = Boolean To (0,1)(Boolean=w1395) -> (0, 1=w1394:i16)
                    }
                    frame #4 {
                      w1499 = 8 ("index")
                      n950 = local read "OH"() -> (w1488:bool[])
                      n951 = local read "BH"() -> (w1489:bool[])
                      n952 = local read "FH"() -> (w1490:bool[])
                      n953 = Split 1D Array(array=w1490, index=w1499) -> (first subarray=w1486:bool[], second subarray=w1487:bool[])
                      n954 = Split 1D Array(array=w1489, index=w1499) -> (first subarray=w1498:bool[], second subarray=w1496:bool[])
                      n955 = Split 1D Array(array=w1488, index=w1499) -> (first subarray=w1497:bool[], second subarray=w1495:bool[])
                      n956 = Build Array(w1486, w1498, w1497) -> (w1485:bool[][])
                      n957 = Build Array(w1487, w1496, w1495) -> (w1484:bool[][])
                      n958 = Or Array Elements(Boolean array=w1485) -> (logical OR=w1493:bool)
                      n959 = Or Array Elements(Boolean array=w1484) -> (logical OR=w1492:bool)
                      n960 = Insert Into Array(array=w1485, new element=w1484) -> (w1483:bool[][])  [unwired: 2 in]
                      n961 = Boolean To (0,1)(Boolean=w1493) -> (0, 1=w1494:i16)
                      n962 = Boolean To (0,1)(Boolean=w1492) -> (0, 1=w1491:i16)
                      n963 = Index Array(array=w1483, index (col) #1=3 ("disabled index (col)"), index (col) #2=4 ("index (col)"), index (col) #3=2 ("index (col)"), index (col) #4=1 ("index (col)"), index (col) #5=6 ("index (col)"), index (col) #6=5 ("index (col)"), index (col) #7=0 ("index (col)"), index (col) #8=7 ("index (col)")) -> (element #1=w1473:bool[], element #2=w1465:bool[], element #3=w1464:bool[], element #4=w1463:bool[], element #5=w1462:bool[], element #6=w1461:bool[], element #7=w1460:bool[], element #8=w1459:bool[])  [unwired: 8 in]
                      n964 = Or Array Elements(Boolean array=w1473) -> (logical OR=w1474:bool)
                      n965 = Or Array Elements(Boolean array=w1464) -> (logical OR=w1470:bool)
                      n966 = Or Array Elements(Boolean array=w1462) -> (logical OR=w1469:bool)
                      n967 = Or Array Elements(Boolean array=w1460) -> (logical OR=w1466:bool)
                      n968 = Or Array Elements(Boolean array=w1465) -> (logical OR=w1472:bool)
                      n969 = Or Array Elements(Boolean array=w1463) -> (logical OR=w1471:bool)
                      n970 = Or Array Elements(Boolean array=w1461) -> (logical OR=w1468:bool)
                      n971 = Or Array Elements(Boolean array=w1459) -> (logical OR=w1467:bool)
                      n972 = Boolean To (0,1)(Boolean=w1474) -> (0, 1=w1458:i16)
                      n973 = Boolean To (0,1)(Boolean=w1470) -> (0, 1=w1456:i16)
                      n974 = Boolean To (0,1)(Boolean=w1469) -> (0, 1=w1454:i16)
                      n975 = Boolean To (0,1)(Boolean=w1466) -> (0, 1=w1452:i16)
                      n976 = Boolean To (0,1)(Boolean=w1472) -> (0, 1=w1457:i16)
                      n977 = Boolean To (0,1)(Boolean=w1471) -> (0, 1=w1455:i16)
                      n978 = Boolean To (0,1)(Boolean=w1468) -> (0, 1=w1453:i16)
                      n979 = Boolean To (0,1)(Boolean=w1467) -> (0, 1=w1451:i16)
                    }
                    frame #5 {
                      n980 = local read "P2 position"() -> (w1514:bool)
                      n981 = local read "P1 position"() -> (w1510:bool)
                      n982 = local read "BH"() -> (w1508:bool[])
                      n983 = local read "OH"() -> (w1509:bool[])
                      n984 = local read "FH"() -> (w1507:bool[])
                      n985 = Or(x="W2", y="E2") -> (x .or. y?=w1518:bool)
                      n986 = Or(x="W1", y="E1") -> (x .or. y?=w1515:bool)
                      n987 = Or Array Elements(Boolean array=w1508) -> (logical OR=w1512:bool)
                      n988 = Or Array Elements(Boolean array=w1509) -> (logical OR=w1513:bool)
                      n989 = Or Array Elements(Boolean array=w1507) -> (logical OR=w1511:bool)
                      n990 = Compound Arithmetic op=OR(w1510, w1511, w1512, w1513, w1514) -> (invert w1517:bool)
                      n991 = And(x=w1517, y=w1518) -> (x .and. y?=w1519:bool)
                      n992 = And(x=w1517, y=w1515) -> (x .and. y?=w1516:bool)
                      n993 = Boolean To (0,1)(Boolean=w1516) -> (0, 1=w1506:i16)
                      n994 = Select(t=2.0, s=w1519, f=w1506) -> (s? t:f=w1501:dbl)
                      n995 = case shown="0, Default" w1501 {
                        tunnel: [w1520 w1549 w1552] -> _
                        frame 0, Default {
                          n996 = local read "coding"() -> (w1520:i32[][])
                        }
                        frame 1 {
                          n997 = local read "W1"() -> (w1543:bool)
                          n998 = local read "W2"() -> (w1544:bool)
                          n999 = local read "P2"() -> (w1521:i32)
                          n1000 = local read "E1"() -> (w1545:bool)
                          n1001 = local read "E2"() -> (w1546:bool)
                          n1002 = local read "P1"() -> (w1547:i32)
                          n1003 = Increment(x=w1521) -> (x+1=w1539:i32)
                          n1004 = Or(x=w1544, y=w1545) -> (x .or. y?=w1541:bool)
                          n1005 = Increment(x=w1547) -> (x+1=w1540:i32)
                          n1006 = Or(x=w1543, y=w1546) -> (x .or. y?=w1542:bool)
                          n1007 = Boolean To (0,1)(Boolean=w1543) -> (0, 1=w1535:i16)
                          n1008 = Boolean To (0,1)(Boolean=w1544) -> (0, 1=w1534:i16)
                          n1009 = Boolean To (0,1)(Boolean=w1545) -> (0, 1=w1529:i16)
                          n1010 = Boolean To (0,1)(Boolean=w1546) -> (0, 1=w1528:i16)
                          n1011 = Select(t=w1539, s=w1541, f=w1521) -> (s? t:f=w1522:i32)
                          n1012 = local read "p1code"() -> (w1537:i32)
                          n1013 = local read "coding"() -> (w1548:i32[][])
                          n1014 = Select(t=w1540, s=w1542, f=w1547) -> (s? t:f=w1524:i32)
                          n1015 = Boolean To (0,1)(Boolean=w1542) -> (0, 1=w1527:i16)
                          n1016 = Boolean To (0,1)(Boolean=w1541) -> (0, 1=w1526:i16)
                          n1017 = local write "P1"(w1524) -> ()
                          n1018 = local write "P2"(w1522) -> ()
                          n1019 = Replace Array Subset(array=w1548, new element #1=w1535, index (row) #1=w1537, index (col) #1=23 ("disabled index (col)"), new element #2=w1534, index (row) #2=w1537, index (col) #2=24 ("disabled index (col)"), new element #3=w1529, index (row) #3=w1537, index (col) #3=25 ("disabled index (col)"), new element #4=w1528, index (row) #4=w1537, index (col) #4=26 ("disabled index (col)"), new element #5=w1527, index (row) #5=w1537, index (col) #5=27 ("disabled index (col)"), new element #6=w1526, index (row) #6=w1537, index (col) #6=28 ("disabled index (col)"), new element #7=w1524, index (row) #7=w1537, index (col) #7=29 ("disabled index (col)"), new element #8=w1522, index (row) #8=w1537, index (col) #8=30 ("disabled index (col)")) -> (w1549:i32[][])
                          n1020 = local write "coding"(w1549) -> ()
                        }
                        frame 2 {
                          n1021 = local read "W1"() -> (w1574:bool)
                          n1022 = local read "W2"() -> (w1575:bool)
                          n1023 = local read "E1"() -> (w1576:bool)
                          n1024 = local read "E2"() -> (w1577:bool)
                          n1025 = Increment(x="P1") -> (x+1=w1571:i32)
                          n1026 = Boolean To (0,1)(Boolean=w1574) -> (0, 1=w1567:i16)
                          n1027 = Boolean To (0,1)(Boolean=w1575) -> (0, 1=w1566:i16)
                          n1028 = Boolean To (0,1)(Boolean=w1576) -> (0, 1=w1561:i16)
                          n1029 = Boolean To (0,1)(Boolean=w1577) -> (0, 1=w1560:i16)
                          n1030 = Or(x=w1574, y=w1577) -> (x .or. y?=w1573:bool)
                          n1031 = Or(x=w1575, y=w1576) -> (x .or. y?=w1572:bool)
                          n1032 = Increment(x="P2") -> (x+1=w1570:i32)
                          n1033 = Select(t=w1570, s=w1572, f="P2") -> (s? t:f=w1554:i32)
                          n1034 = Select(t=w1571, s=w1573, f="P1") -> (s? t:f=w1556:i32)
                          n1035 = Boolean To (0,1)(Boolean=w1573) -> (0, 1=w1559:i16)
                          n1036 = Boolean To (0,1)(Boolean=w1572) -> (0, 1=w1558:i16)
                          n1037 = local read "p2code"() -> (w1553:i32)
                          n1038 = local read "coding"() -> (w1578:i32[][])
                          n1039 = local write "P1"(w1556) -> ()
                          n1040 = Replace Array Subset(array=w1578, new element #1=w1567, index (row) #1=w1553, index (col) #1=23 ("disabled index (col)"), new element #2=w1566, index (row) #2=w1553, index (col) #2=24 ("disabled index (col)"), new element #3=w1561, index (row) #3=w1553, index (col) #3=25 ("disabled index (col)"), new element #4=w1560, index (row) #4=w1553, index (col) #4=26 ("disabled index (col)"), new element #5=w1559, index (row) #5=w1553, index (col) #5=27 ("disabled index (col)"), new element #6=w1558, index (row) #6=w1553, index (col) #6=28 ("disabled index (col)"), new element #7=w1556, index (row) #7=w1553, index (col) #7=29 ("disabled index (col)"), new element #8=w1554, index (row) #8=w1553, index (col) #8=30 ("disabled index (col)")) -> (w1552:i32[][])
                          n1041 = local write "P2"(w1554) -> ()
                          n1042 = local write "coding"(w1552) -> ()
                        }
                      }
                    }
                    frame #6 {
                      w1579 = i16 0
                      n1043 = Boolean To (0,1)(Boolean="S1") -> (0, 1=w1585:i16)
                      n1044 = Boolean To (0,1)(Boolean="S2") -> (0, 1=w1584:i16)
                      n1045 = Boolean To (0,1)(Boolean="1") -> (0, 1=w1583:i16)
                      n1046 = Boolean To (0,1)(Boolean="2") -> (0, 1=w1582:i16)
                      n1047 = Boolean To (0,1)(Boolean="3") -> (0, 1=w1581:i16)
                      n1048 = Boolean To (0,1)(Boolean="4") -> (0, 1=w1580:i16)
                    }
                    frame #7 {
                      w1593 = FALSE ("4 6")
                      n1049 = local write "1 6"(w1593) -> ()
                      n1050 = local write "2 6"(w1593) -> ()
                      n1051 = local write "3 6"(w1593) -> ()
                      n1052 = local write "4 6"(w1593) -> ()
                      n1053 = local write "5 6"(w1593) -> ()
                      n1054 = local write "6 6"(w1593) -> ()
                      n1055 = local write "7 6"(w1593) -> ()
                      n1056 = local write "8 6"(w1593) -> ()
                      n1057 = local write "1 5"(w1593) -> ()
                      n1058 = local write "2 5"(w1593) -> ()
                      n1059 = local write "3 5"(w1593) -> ()
                      n1060 = local write "4 5"(w1593) -> ()
                      n1061 = local write "5 5"(w1593) -> ()
                      n1062 = local write "6 5"(w1593) -> ()
                      n1063 = local write "7 5"(w1593) -> ()
                      n1064 = local write "8 5"(w1593) -> ()
                      n1065 = local write "1 4"(w1593) -> ()
                      n1066 = local write "2 4"(w1593) -> ()
                      n1067 = local write "3 4"(w1593) -> ()
                      n1068 = local write "4 4"(w1593) -> ()
                      n1069 = local write "5 4"(w1593) -> ()
                      n1070 = local write "6 4"(w1593) -> ()
                      n1071 = local write "7 4"(w1593) -> ()
                      n1072 = local write "8 4"(w1593) -> ()
                      n1073 = local write "1 3"(w1593) -> ()
                      n1074 = local write "2 3"(w1593) -> ()
                      n1075 = local write "3 3"(w1593) -> ()
                      n1076 = local write "4 3"(w1593) -> ()
                      n1077 = local write "5 3"(w1593) -> ()
                      n1078 = local write "6 3"(w1593) -> ()
                      n1079 = local write "7 3"(w1593) -> ()
                      n1080 = local write "8 3"(w1593) -> ()
                      n1081 = local write "1 2"(w1593) -> ()
                      n1082 = local write "2 2"(w1593) -> ()
                      n1083 = local write "3 2"(w1593) -> ()
                      n1084 = local write "4 2"(w1593) -> ()
                      n1085 = local write "5 2"(w1593) -> ()
                      n1086 = local write "6 2"(w1593) -> ()
                      n1087 = local write "7 2"(w1593) -> ()
                      n1088 = local write "8 2"(w1593) -> ()
                      n1089 = local write "1"(w1593) -> ()
                      n1090 = local write "2"(w1593) -> ()
                      n1091 = local write "3"(w1593) -> ()
                      n1092 = local write "4"(w1593) -> ()
                      n1093 = local write "5"(w1593) -> ()
                      n1094 = local write "6"(w1593) -> ()
                      n1095 = local write "7"(w1593) -> ()
                      n1096 = local write "8"(w1593) -> ()
                      n1097 = local write "BL 3"(w1593) -> ()
                      n1098 = local write "BL 2"(w1593) -> ()
                      n1099 = local write "BM 3"(w1593) -> ()
                      n1100 = local write "BM 2"(w1593) -> ()
                      n1101 = local write "BR 2"(w1593) -> ()
                      n1102 = local write "BR 3"(w1593) -> ()
                      n1103 = local write "W1"(w1593) -> ()
                      n1104 = local write "W2"(w1593) -> ()
                      n1105 = local write "E1"(w1593) -> ()
                      n1106 = local write "E2"(w1593) -> ()
                      n1107 = local write "TL 3"(w1593) -> ()
                      n1108 = local write "TL 2"(w1593) -> ()
                      n1109 = local write "TM 2"(w1593) -> ()
                      n1110 = local write "TM 3"(w1593) -> ()
                      n1111 = local write "TR 2"(w1593) -> ()
                      n1112 = local write "TR 3"(w1593) -> ()
                      n1113 = local write "S1"(w1593) -> ()
                      n1114 = local write "S2"(w1593) -> ()
                      n1115 = local write "1"(w1593) -> ()
                      n1116 = local write "2"(w1593) -> ()
                      n1117 = local write "3"(w1593) -> ()
                      n1118 = local write "4"(w1593) -> ()
                      n1119 = local read "coding"() -> (w1592:i32[][])
                      n1120 = local write "CL 3"(w1593) -> ()
                      n1121 = local write "CL 2"(w1593) -> ()
                      n1122 = local write "CM 2"(w1593) -> ()
                      n1123 = local write "CM 3"(w1593) -> ()
                      n1124 = local write "CR  2"(w1593) -> ()
                      n1125 = local write "CR  3"(w1593) -> ()
                    }
                  }
                  n1126 = call "IMAQ Dispose"("Image"=w1225) -> ()  [unwired: 5 in, 1 out]
                  n1127 = Build Array(w1241, w1242, w1281, w1280, w1279, w1278, w1277, w1276, w1270, w1275, w1274, w1273, w1272, w1271, w1269, w1268, w1267, w1266, w1265, w1264, w1263, w1262, w1261, w1260, w1259, w1258, w1257, w1256, w1255, w1254, w1253, w1252, w1251, w1250, w1249, w1248, w1247, w1246, w1245) -> (w1233:i32[])
                  n1128 = Delete From Array(array=w1233, index=0) -> (array with subset deleted=w1231:i32[])  [unwired: 1 in, 1 out]
                  n1129 = Insert Into Array(array=w1227, new element=w1233) -> (w1228:i32[][])  [unwired: 2 in]
                  n1130 = Array Max & Min(array=w1231) -> (max value=w1230:i32)  [unwired: 3 out]
                  n1131 = Equal To 0?(x=w1230) -> (x = 0?=w1229:bool)
                  n1132 = Select(t=w1227, s=w1229, f=w1228) -> (s? t:f=w1226:i32[][])
                  n1133 = Index Array(array=w1226, index (col)=0 ("disabled index (col)")) -> (element=w1235:i32[])  [unwired: 1 in]
                  n1134 = Array Max & Min(array=w1235) -> (max value=→"Last coded":i32)  [unwired: 3 out]
                  n1135 = local write "coding"(w1226) -> ()
                }
              }
              n1136 = case shown="True" "Stop and save" {
                tunnel: [FALSE ("T button?") w1090] -> w1055
                frame False {
                }
                frame True {
                  n1137 = Two Button Dialog(message="You are about to stop the notation process", 2:"Stop and Save" ("Left Button Text (\"Yes\")")) -> (T button?=w1090:bool)  [unwired: 1 in]
                }
              }
              n1138 = Strip Path(path="Save data") -> (stripped path=w1066:path)  [unwired: 1 out]
              n1139 = call <vilib>:"Get File Extension.vi"("file"="Save data") -> ("filename without extension"=w1069:string)  [unwired: 7 in, 3 out]
              n1140 = Path To String(path=w1066) -> (string=w1065:string)
              n1141 = Concatenate Strings(w1065, "\\" ("string"), w1069, "(BStAT DATA).xls" ("string")) -> (w1064:string)
              n1142 = String To Path(string=w1064) -> (path=w1061:path)
              n1143 = call <vilib>:"Check if File or Folder Exists.vi"("path"=w1061) -> ("file or folder exists?"=w1062:bool)  [unwired: 8 in, 2 out]
            }
            n1144 = local read "F_frame"() -> (w1035:u32)
            n1145 = local read "S_frame"() -> (w1034:u32)
            n1146 = property on="Progress..." class="Slide (strict)"("Scale.Maximum"=w1035, "Scale.Minimum"=w1034, "Visible"=w1019) -> ()  [unwired: 2 in, 2 out]
            n1147 = Not(x=w1019) -> (.not. x?=w1020:bool)
            n1148 = property on="Drag control" class="Slide (strict)"("Visible"=w1020) -> ()  [unwired: 2 in, 2 out]
            n1149 = Path to Array of Strings(0:w1029) -> (2:w1030:string[])  [unwired: 1 out]
            n1150 = Array Size(array=w1030) -> (size(s)=w1031:i32)
            n1151 = Decrement(x=w1031) -> (x-1=w1032:i32)
            n1152 = Index Array(array=w1030, index=w1032) -> (element=w1028:string)
            n1153 = call "EVENTS(SubVI).vi"() -> ("Events"=w1026:string)  [unwired: 1 in]
            n1154 = Concatenate Strings("avi file" ("string"), w1025, w1028, w1025, w1025, w1026) -> (w1027:string)
            n1155 = call "IMAQ AVI Close"("Avi Refnum"=w1023) -> ()  [unwired: 10 in, 1 out]
            n1156 = case shown="False" w1017 {
              tunnel: w1018 -> [w1048 w1050]
              tunnel: w1027 -> [w1045 _]
              tunnel: w1016 -> [w1043 w1049]
              frame False {
                n1157 = Open/Create/Replace File(file path (use dialog)=w1043, operation (0:open)=T3."create") -> (refnum out=w1046:refnum<file>)  [unwired: 4 in, 2 out]
                n1158 = Write to Text File(file (use dialog)=w1046, text=w1045) -> (refnum out=w1042:refnum<file>)  [unwired: 2 in, 2 out]
                n1159 = Close File(refnum=w1042) -> (path=w1041:path)  [unwired: 1 in, 1 out]
                n1160 = call-poly <vilib>:"Write To Spreadsheet File.vi"("append to file? (new file:F)"=TRUE, "2D data"=w1048, "file path (dialog if empty)"=w1041) -> ()  [unwired: 5 in, 1 out]
              }
              frame True {
                n1161 = call-poly <vilib>:"Write To Spreadsheet File.vi"("append to file? (new file:F)"=TRUE, "2D data"=w1050, "file path (dialog if empty)"=w1049) -> ()  [unwired: 5 in, 1 out]
              }
            }
            n1162 = property on="playback speed" class="Slide (strict)"("Visible"=w1022) -> ()  [unwired: 2 in, 2 out]
            n1163 = property on="Progress..." class="Slide (strict)"("Visible"=w1022) -> ()  [unwired: 2 in, 2 out]
            n1164 = property on="UNDO" class="Bool (strict)"("Visible"=w1022) -> ()  [unwired: 2 in, 2 out]
            n1165 = property on="Last coded" class="DigNum (strict)"("Visible"=w1022) -> ()  [unwired: 2 in, 2 out]
            n1166 = property on="Last coded" class="DigNum (strict)"("Visible"=w1021) -> ()  [unwired: 2 in, 2 out]
            n1167 = property on="UNDO" class="Bool (strict)"("Visible"=w1021) -> ()  [unwired: 2 in, 2 out]
            n1168 = property on="playback speed" class="Slide (strict)"("Visible"=w1021) -> ()  [unwired: 2 in, 2 out]
            "coding" <- i32[][] [] ("coding")
          }
        }
        "S_frame" <- w976
        "F_frame" <- w976
      }
    }
  }
